vi "Measure vs B2Dv9.vi"() -> ()   [LabVIEW 2009]
doc: "This VI is an example operator panel.\n\nThe VI contains a table for the field values that may be configured manually, or loaded by checking the \"Prompt for File\" box. The data file should contain 3 columns of data, with each column delimited by a tab character.\n\nBefore the VI is executed, set the desired field units and coordinate system. Once the VI is started, follow the directions in the STATUS indicator to operate. Once a field value is achieved, it will be held indefinitely with no user intervention.\n\nThe present field is displayed in the selected units and coordinate system. The present field is queried once per second.\n\nIf a field point is specified that is outside the limits for the magnet, the VI will abort execution."
uses:
  <vilib>/Utility/file.llb/Read From Spreadsheet File (DBL).vi
panel:
  in  "go to zero at end of measurement":bool=TRUE
  in  "AH (2500)":bool=TRUE
  out "fieldvalues":string[](array[string])=["0.5", "91"]
  in  "Nr. of Accumulations":i32=3
  out "appended array":dbl[](array[numeric])=[3.9998302517106903, 162.36209894569686, 0.0, 0.0, 0.0, 0.0, 0.0, 0.0, 0.0, 0.0, 13.342744999999999, 0.0, 0.0, 3409919392.4083776]
  in  "X Axis":enum16{"B", "phi"}(ring)=enum."phi"
  in  "Y Axis":T1(ring)=enum."HP (V)"
  out "XY Graph":T2(graph)={"measured data"=[130.77697934473076, 131.17238359064999, 131.57493282279165, 131.97089096284472, 132.3709005627829, 132.7747269835502, 133.17115299337118, 133.57699453159358, 133.97291907281786, 134.37163450772164, 134.7728190578919, 135.17563033959266, 135.57333372461295, 135.97830344291987, 136.37202071047088, 136.77617688548457, 137.17728611854096, 137.57344246367185, 137.96927398938195, 138.37484712631183, 138.7678966828463, 139.1744152195974, 139.5694101008014, 139.9620548045032, 140.3756352936819, 140.76443013035026, 141.1688823561444, 141.56815184223575, 141.9675976417151, 142.3659953584458, 142.775676716873, 143.16379154430956, 143.57809589273134, 143.96940395419173, 144.37063731617485, 144.76393855420042, 145.16100725100878, 145.5613313376955, 145.9608116195239, 146.37481274459287, 146.76791709360782, 147.16896149127172, 147.5663143604346, 147.9678028289989, 148.36962760092925, 148.76598884997566, 149.16767338072717, 149.56607764958403, 149.95999407346423, 150.3722468362733, 150.76361618206533, 151.15525055318153, 151.57358356130908, 151.9672547235955, 152.360163563412, 152.76137159791082, 153.15948892689605, 153.56793804327447, 153.9626908891637, 154.35791457944399, 154.76495537165297, 155.1633906497064, 155.56156935652382, 155.96111561211768, 156.36610319740612, 156.76559958179956, 157.17093878264262, 157.56689125105595, 157.96437052200662, 158.376205209266, 158.76161261329872, 159.16724590816438, 159.55971274891448, 159.96783078495864, 160.36059978391282, 160.75915896709176, 161.17541940848784, 161.56387349300712, 161.96414973052572, 162.36209894569686], "measured data"=[47.8127675, 47.3142275, 46.9315925, 46.6304225, 46.0396825, 45.6777125, 45.4570175, 45.070972499999996, 44.789265, 44.3558025, 43.6591325, 43.409885, 43.162465, 42.71473, 42.531679999999994, 42.226214999999996, 41.899212500000004, 41.3661625, 41.03545, 40.637135, 40.367885, 40.046705, 39.865300000000005, 39.57427, 39.035422499999996, 38.758669999999995, 38.5814575, 38.362825, 37.764005, 37.63395250000001, 37.1175925, 15.572479999999999, -4.558832499999999, -4.02452, 18.98894, -4.1475925, -5.032675, 25.0248675, 27.1825925, 28.551062500000004, 27.772665, 26.5350725, 23.5985575, 27.104, 24.8567975, 23.797494999999998, 25.486569999999997, 24.9155175, 26.26794, 24.482997499999996, 25.039457499999997, 13.34384, 13.3442075, 13.3447275, 13.34462, 13.344155, 54.256817500000004, 13.3434, 13.3445175, 13.343632500000002, 13.3429575, 13.343734999999999, 13.3441525, -7.896862499999999, 13.344205, -8.8820475, 13.343815, 13.3419875, -24.604432499999998, 13.342722499999999, -6.686962499999998, 13.34337, 13.343815, 13.344335000000001, -23.786430000000003, 13.34392, 13.343657499999999, 13.3431125, 13.3426425, 13.342744999999999]}
  in  "GPIB HP 2":string="13"
  in  "Wait between \nVectors":bool=TRUE
  in  "Change\nPID\n(polar coordinates)":bool
  in  "Wait between \nVectors (ms)":u32=4000
  out "measured data":dbl[][](array[numeric])
  in  "Notes:":string="Datum: 6.04.12, Uhrzeit: 12:30,  T 4K,Winkelsweep 1° Winkelschritte, warten bei jedem Feldpunkt (measurevsB2Dv9.vi))4s, vectorsm1.txt, praktikumsprobenstab, Sweep  0.15, CrB auf CuBe Sensoren" caption="Notizen:"
  out "Messfile Refnum":refnum<file>
  in  "Measurement File":path=path "D:/UserData/Matthias/Messungen/CrB/120406/CrB_120406_anglesweep4K1.txt"
  in  "Sample name:":string="CrB"
  in  "HP 1":bool
  in  "GPIB HP":string="14"
  in  "HP 2":bool
  in  "LI 3":bool
  in  "GPIB L 3":string="8"
  in  "LI 2":bool
  in  "GPIB L 2":string="8"
  in  "LI 1":bool
  in  "GPIB L 1":string="8"
  out "Number of lines":i32=2
  in  "Operation":u16(ring)=1 items=["Stepwise", "Continous"]
  out "Ramp Rate along Vector (T/min)":dbl=0.15 format="%.3f"
  out "Current Ramp Rate Z (T/min)":dbl=0.015702717677741673 format="%.3f"
  out "Current Ramp Rate Y (T/min)":dbl=0.1491758179382072 format="%.3f"
  in  "User defined Ramp Rate (T/min)":bool=TRUE
  in  "User defined Ramp Rate (T/min)":dbl=0.15 format="%.3f"
  in  "Z-Axis Communications Config":T3={"GPIB address"=22, "GPIB bus"=1, "connection ID"=refnum, "IP"="111.111.111.1", "Active Comm Interface"=0, "Serial Port"="", "Programmer Type"=0} {"Programmer Type" items=["Model 430", "Model 420"]; "Active Comm Interface" items=["TCP/IP (Model 430 Only)", "RS232", "IEEE488"]}
  in  "Max Ramp Rate - Y Axis (A/s)":dbl=0.055 format="%.3f"
  in  "Max Ramp Rate - Z Axis (A/s)":dbl=0.19 format="%.3f"
  in  "Magnitude Limit (kG)":dbl=45.1 format="%.3f"
  in  "Y-Axis Communications Config":T3={"GPIB address"=22, "GPIB bus"=1, "connection ID"=refnum, "IP"="111.111.111.2", "Active Comm Interface"=0, "Serial Port"="", "Programmer Type"=0} {"Programmer Type" items=["Model 430", "Model 420"]; "Active Comm Interface" items=["TCP/IP (Model 430 Only)", "RS232", "IEEE488"]}
  out "Cartesian Display (T)":T4={"Y-Axis Field (T)"=0.01746, "Z-Axis Field (T)"=0.99986} {"Z-Axis Field (T)" format="%.3f"; "Y-Axis Field (T)" format="%.3f"}
  in  "Starting index":i32=1
  in  "Normal color":u32(colorbox)=11711154
  in  "Highlight color":u32(colorbox)=16711680
  in  "Prompt for File?":bool
  out "Continue Execution?":bool=TRUE
  out "error out":T5
  in  "error in":T5
  out "STATUS":string="Ramping to field vector 1..."
  in  "Ramping Control":u16(ring)=1 items=["NEXT VECTOR", "RAMPING", "HOLDING", "PAUSE", "ZERO"]
  out "Cartesian Display (kG)":T6 {"Z-Axis Field (kG)" format="%.3f"; "Y-Axis Field (kG)" format="%.3f"}
  in  "Field Values":string[][](table)=[["0.5", "90"], ["0.5", "91"]]
  out "Switch Heaters":bool=TRUE
  out "Polar Display (T)":T7={"q (degrees)"=89.97708168941708, "Field Magnitude (T)"=0.5000000399999984} {"Field Magnitude (T)" format="%.3f"; "q (degrees)" format="%.3f"}
  out "Polar Display (kG)":T8 {"Field Magnitude (kG)" format="%.3f"; "q (degrees)" format="%.3f"}
  in  "Coordinate System":u16(ring)=1 items=["Cartesian", "Polar"]
  in  "Magnetic Field Units":u16(ring)=1 items=["kG", "Tesla"]
  # "Punkt für Punkt Messung, gotozero am Ende der Messung und switch heater off"
  # "Measurement Display"
  # "Measurement Settings"
  # "Magnet Settings"
  # "Max Ramp Rate z: 1.27 T/min\nMax Ramp Rate y: 0.17 T/min"
  # "Devices"
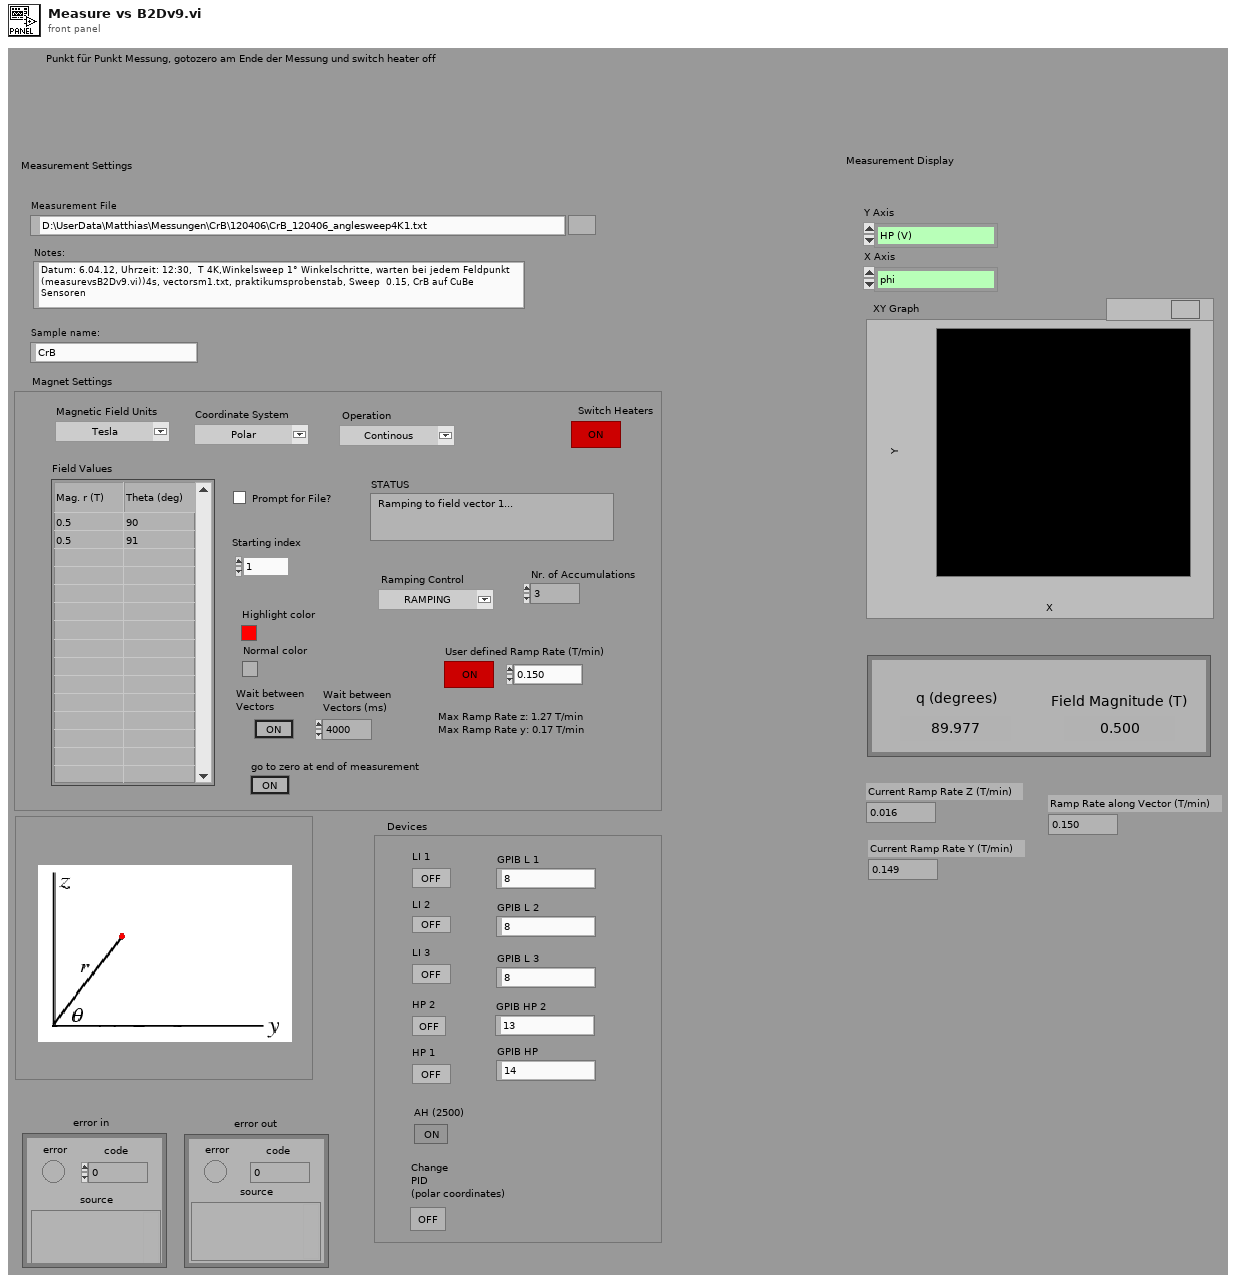
[diagram p1: front panel]
types:
  T1 = enum16{"B", "phi", "LI 1 Vx", "LI 1 phase", "LI 2 Vx", "LI 2 phase", "LI 3 Vx", "LI 3 phase", "LI 4 Vx", "LI 4 phase", "HP (V)", "AH C (pF)", "AH loss"}
  T2 = cluster{"measured data":dbl[], "measured data":dbl[]}
  T3 = cluster{"GPIB address":i16, "GPIB bus":i16, "connection ID":refnum<k5>, "IP":string, "Active Comm Interface":u16, "Serial Port":refnum<visa-resource-name>, "Programmer Type":u16}
  T4 = cluster{"Y-Axis Field (T)":dbl, "Z-Axis Field (T)":dbl}
  T5 = cluster{"error":bool, "code":i32, "source":string}
  T6 = cluster{"Y-Axis Field (kG)":dbl, "Z-Axis Field (kG)":dbl}
  T7 = cluster{"q (degrees)":dbl, "Field Magnitude (T)":dbl}
  T8 = cluster{"q (degrees)":dbl, "Field Magnitude (kG)":dbl}
  T9 = enum16{"", "RAMPING", "HOLDING", "PAUSED", "MANUAL UP", "MANUAL DOWN", "ZEROING CURRENT", "QUENCH DETECTED", "HEATING SWITCH"}
  T10 = enum16{"", "RAMPING", "HOLDING", "PAUSED", "MANUAL UP", "MANUAL DOWN", "ZEROING CURRENT", "QUENCH DETECTED", "HEATING SWITCH", "AT ZER0", "COOLING SWITCH"}
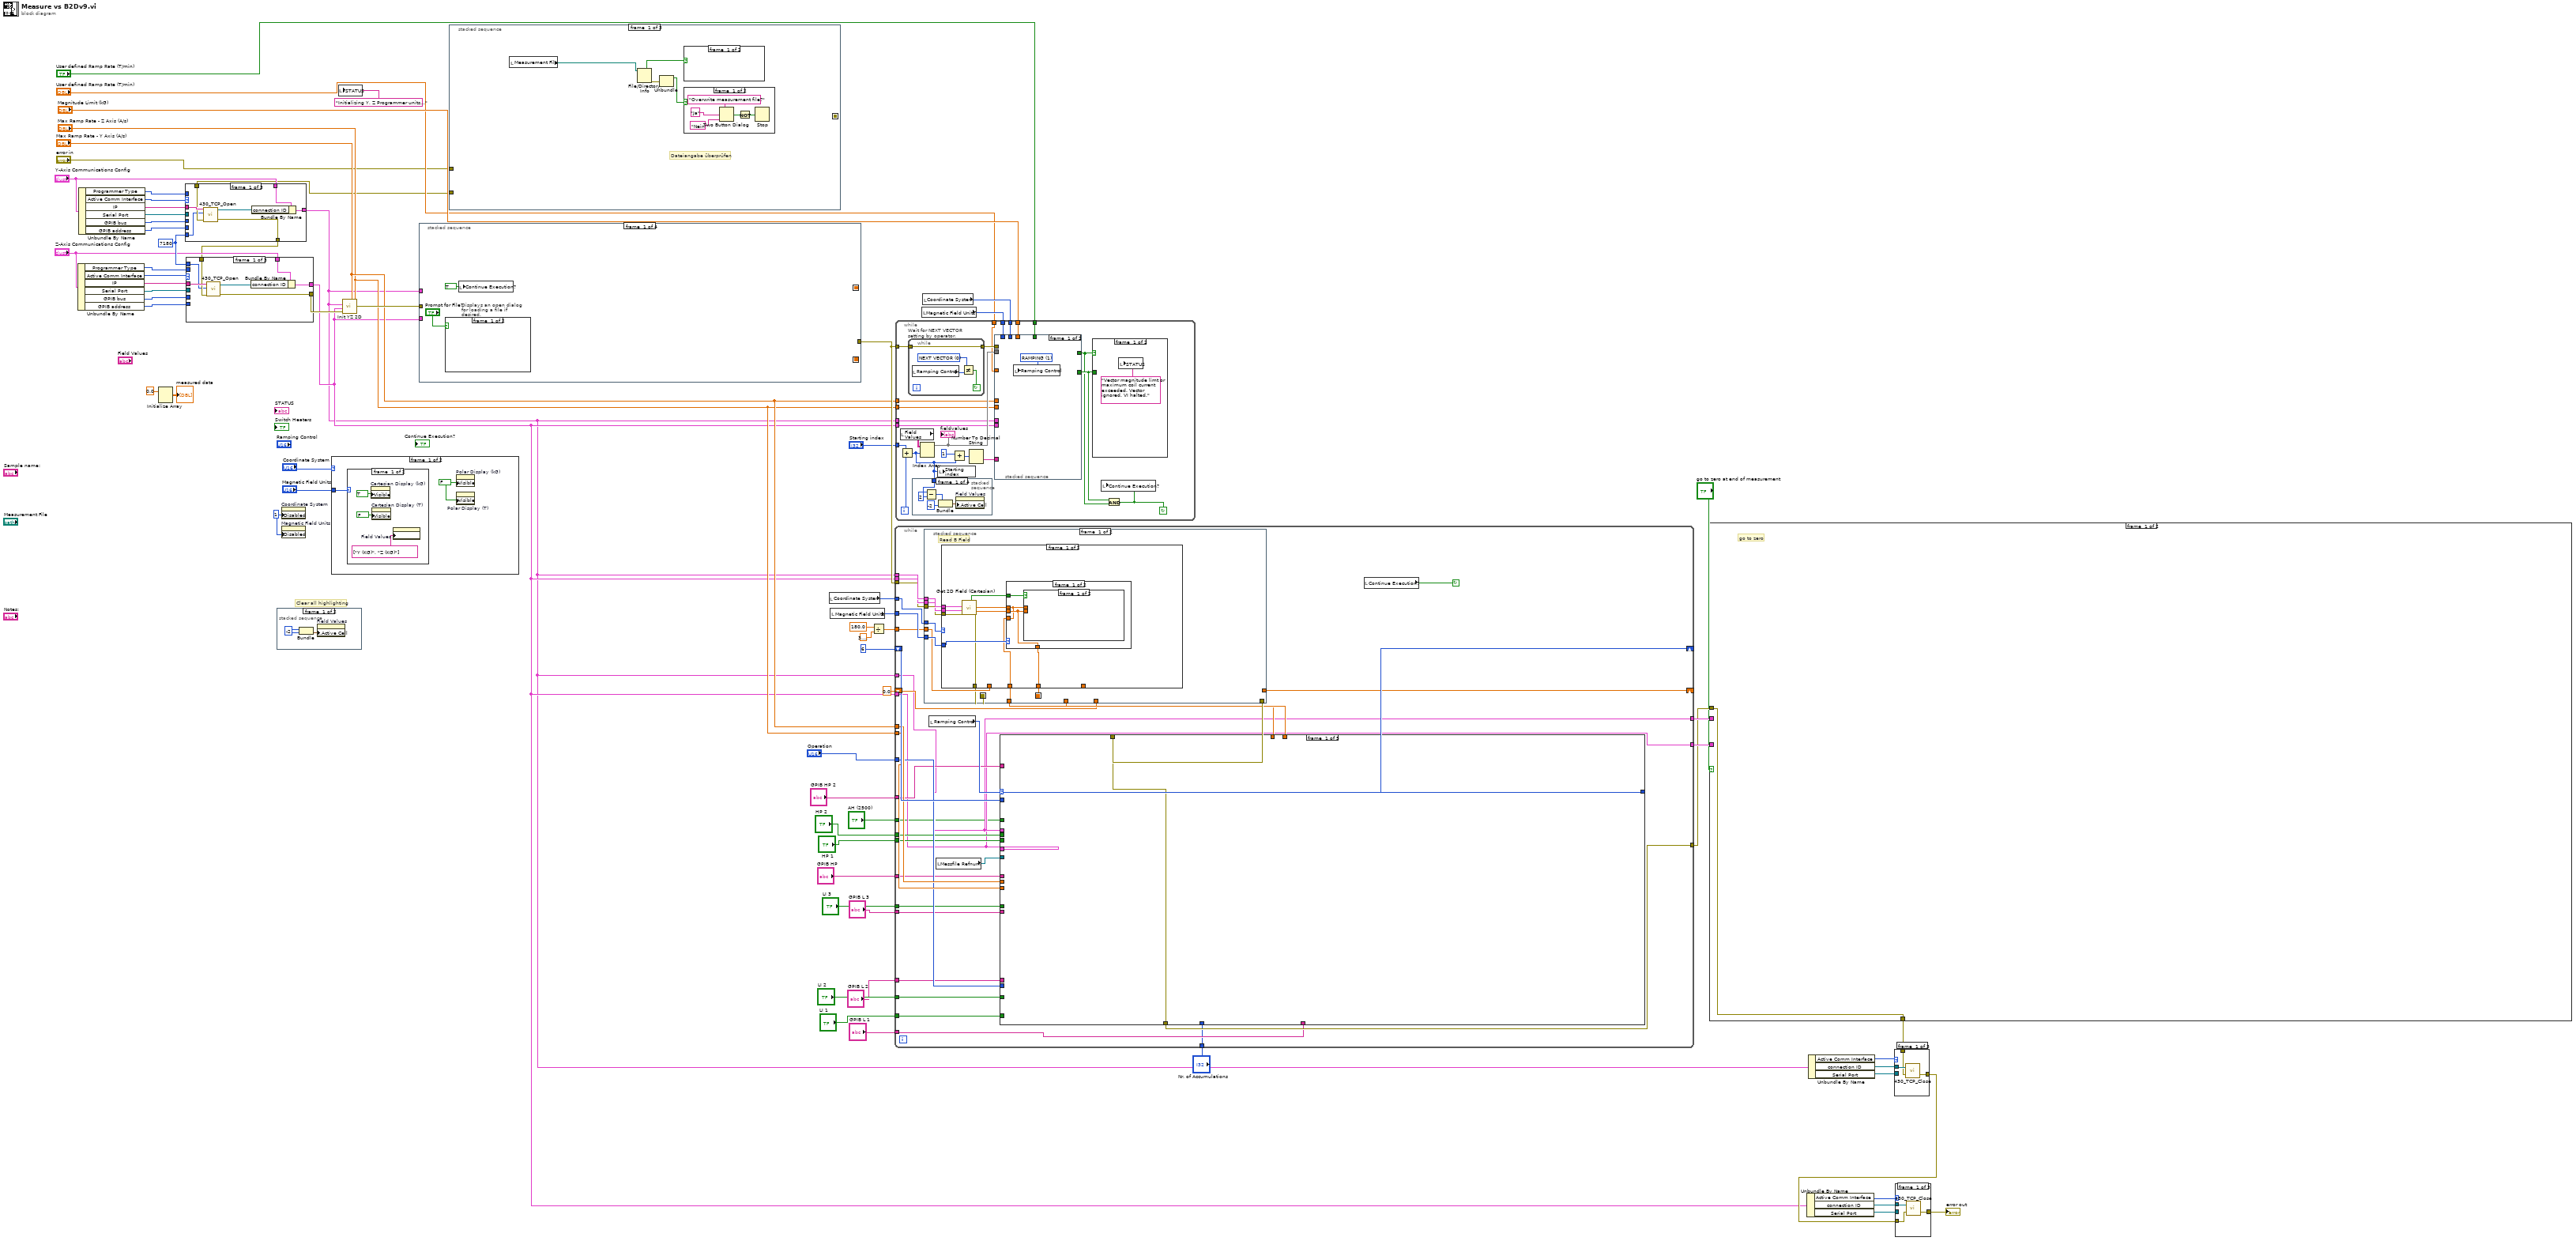
[diagram p0: block diagram]
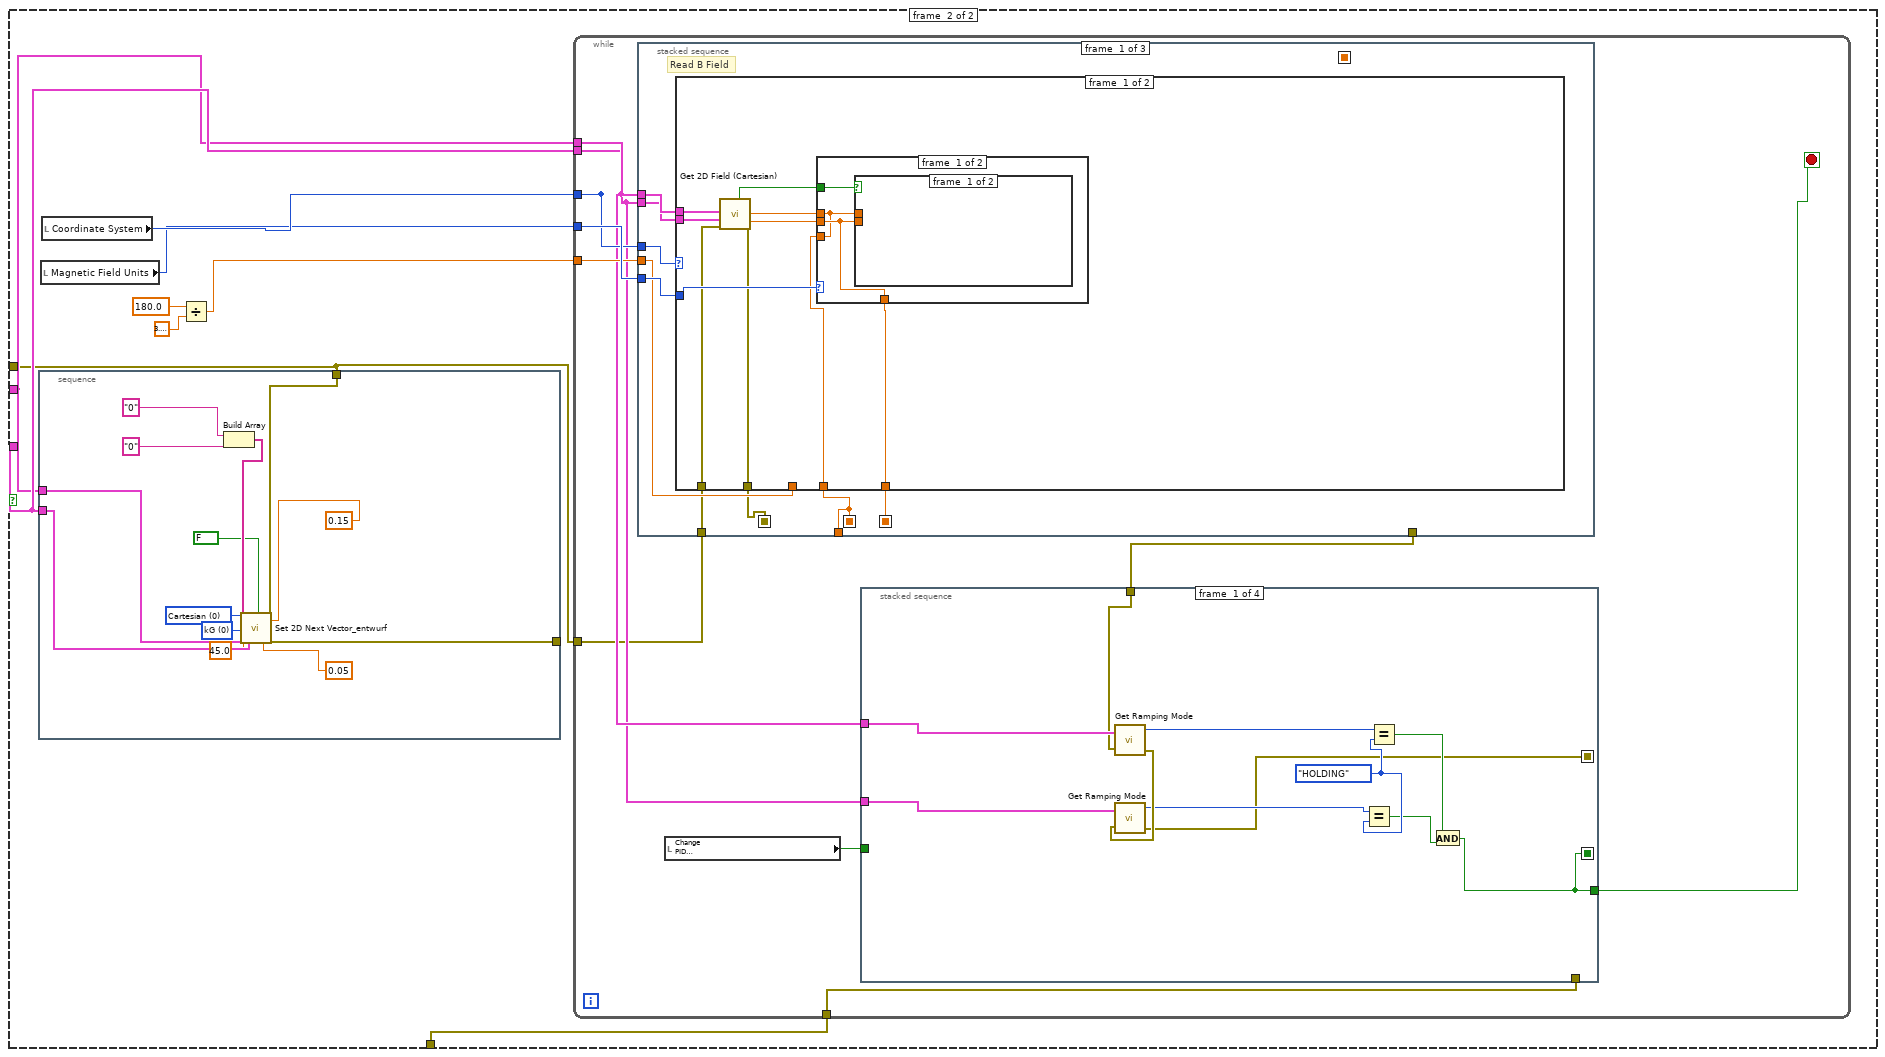
[diagram p2: hidden frame]
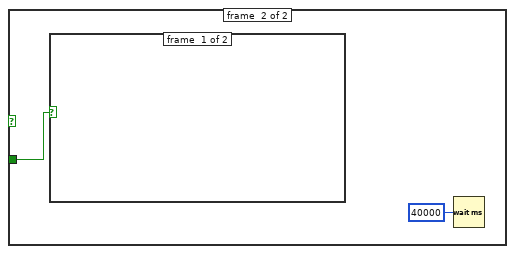
[diagram p4: hidden frame]
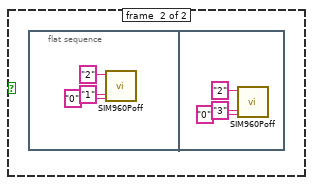
[diagram p5: hidden frame]
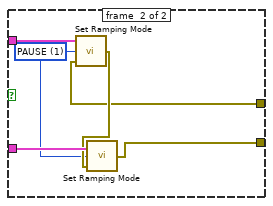
[diagram p7: hidden frame]
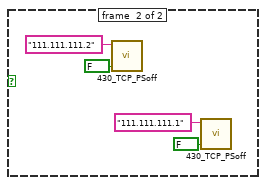
[diagram p9: hidden frame]
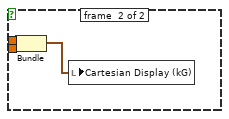
[diagram p10: hidden frame]
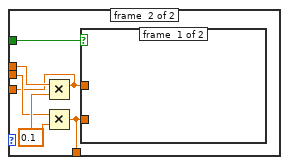
[diagram p11: hidden frame]
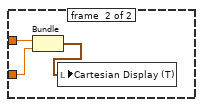
[diagram p12: hidden frame]
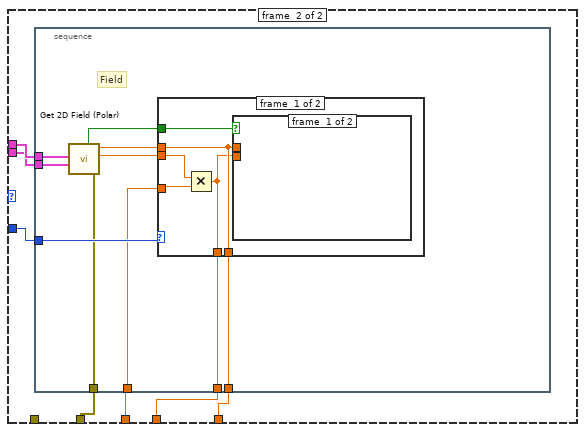
[diagram p13: hidden frame]
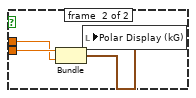
[diagram p14: hidden frame]
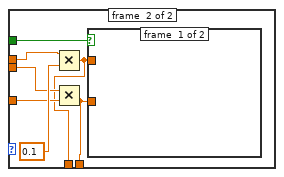
[diagram p15: hidden frame]
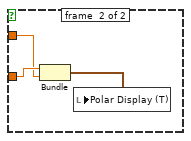
[diagram p16: hidden frame]
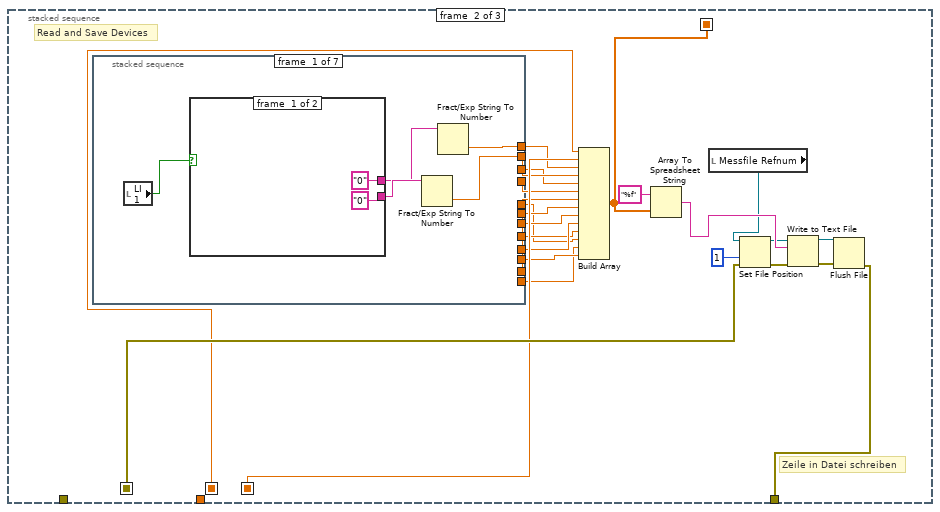
[diagram p17: hidden frame]
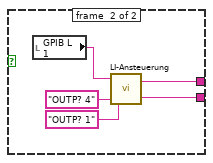
[diagram p18: hidden frame]
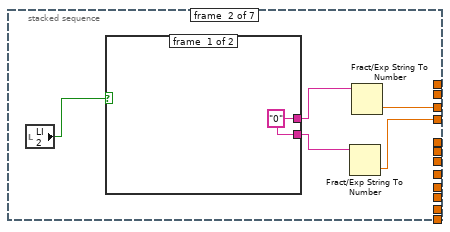
[diagram p19: hidden frame]
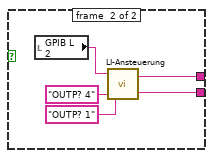
[diagram p20: hidden frame]
diagram:
  w55 = 7180 ("TCP Port")
  w68 = u8 1 ("Write Attribute")
  # "Clear all highlighting"
  n1 = Unbundle By Name("Z-Axis Communications Config") -> ("Programmer Type"=w34:u16, "Active Comm Interface"=w54:u16, "IP"=w51:string, "Serial Port"=w50:refnum<visa-resource-name>, "GPIB bus"=w33:i16, "GPIB address"=w32:i16)
  n2 = Unbundle By Name("Y-Axis Communications Config") -> ("Programmer Type"=w28:u16, "Active Comm Interface"=w53:u16, "IP"=w52:string, "Serial Port"=w49:refnum<visa-resource-name>, "GPIB bus"=w29:i16, "GPIB address"=w30:i16)
  n3 = Initialize Array(0.0 ("element")) -> (→"measured data":dbl[][])  [unwired: 2 in]
  n4 = stacked-sequence {
    frame #0 {
      w71 = -2
      n5 = Bundle(w71, w71) -> (w72:cluster{i32, i32})  [unwired: 1 in]
      n6 = property on="Field Values" class="Tbl (strict)"("Active Cell:Active Cell"=w72) -> ()  [unwired: 2 in, 2 out]
    }
    frame #1 {
      n7 = property on="Field Values" class="Tbl (strict)"("Active Cell:Cell Background Color"="Normal color") -> ()  [unwired: 2 in, 2 out]
    }
  }
  n8 = property on="Coordinate System" class="Ring (strict)"("Disabled"=w68) -> ()  [unwired: 2 in, 2 out]
  n9 = property on="Magnetic Field Units" class="Ring (strict)"("Disabled"=w68) -> ()  [unwired: 2 in, 2 out]
  n10 = case shown="0, Default" "Coordinate System" {
    tunnel: "Magnetic Field Units" -> [w75 w83]
    frame #0 {
      w74 = FALSE ("Write Attribute")
      (unwired) FALSE ("Write Attribute")
      (unwired) TRUE ("Write Attribute")
      n11 = case shown="1" w75 {
        frame #0 {
          n12 = property on="Cartesian Display (kG)" class="Cluster (strict)"("Visible"=TRUE ("Write Attribute")) -> ()  [unwired: 2 in, 2 out]
          n13 = property on="Cartesian Display (T)" class="Cluster (strict)"("Visible"=FALSE ("Write Attribute")) -> ()  [unwired: 2 in, 2 out]
          n14 = property on="Field Values" class="Tbl (strict)"("Column Header Strings[]"=string[] ["Y (KG)", "Z (KG)"] ("Write Attribute")) -> ()  [unwired: 2 in, 2 out]
        }
        frame #1 {
          n15 = property on="Cartesian Display (kG)" class="Cluster (strict)"("Visible"=FALSE ("Write Attribute")) -> ()  [unwired: 2 in, 2 out]
          n16 = property on="Cartesian Display (T)" class="Cluster (strict)"("Visible"=TRUE ("Write Attribute")) -> ()  [unwired: 2 in, 2 out]
          n17 = property on="Field Values" class="Tbl (strict)"("Column Header Strings[]"=string[] ["Y (T)", "Z (T)"] ("Write Attribute")) -> ()  [unwired: 2 in, 2 out]
        }
      }
      n18 = property on="Polar Display (kG)" class="Clust (strict)"("Visible"=w74) -> ()  [unwired: 2 in, 2 out]
      n19 = property on="Polar Display (T)" class="Clust (strict)"("Visible"=w74) -> ()  [unwired: 2 in, 2 out]
    }
    frame #1 {
      (unwired) FALSE ("Write Attribute")
      (unwired) TRUE ("Write Attribute")
      w82 = FALSE ("Write Attribute")
      n20 = case shown="1" w83 {
        frame #0 {
          n21 = property on="Polar Display (kG)" class="Clust (strict)"("Visible"=TRUE ("Write Attribute")) -> ()  [unwired: 2 in, 2 out]
          n22 = property on="Polar Display (T)" class="Clust (strict)"("Visible"=FALSE ("Write Attribute")) -> ()  [unwired: 2 in, 2 out]
          n23 = property on="Field Values" class="Tbl (strict)"("Column Header Strings[]"=string[] ["Mag. r (KG)", "Theta (deg)"] ("Write Attribute")) -> ()  [unwired: 2 in, 2 out]
        }
        frame #1 {
          n24 = property on="Polar Display (kG)" class="Clust (strict)"("Visible"=FALSE ("Write Attribute")) -> ()  [unwired: 2 in, 2 out]
          n25 = property on="Polar Display (T)" class="Clust (strict)"("Visible"=TRUE ("Write Attribute")) -> ()  [unwired: 2 in, 2 out]
          n26 = property on="Field Values" class="Tbl (strict)"("Column Header Strings[]"=string[] ["Mag. r (T)", "Theta (deg)"] ("Write Attribute")) -> ()  [unwired: 2 in, 2 out]
        }
      }
      n27 = property on="Cartesian Display (kG)" class="Cluster (strict)"("Visible"=w82) -> ()  [unwired: 2 in, 2 out]
      n28 = property on="Cartesian Display (T)" class="Cluster (strict)"("Visible"=w82) -> ()  [unwired: 2 in, 2 out]
    }
  }
  n29 = local write "STATUS"("Initializing Y, Z Programmer units..." ("STATUS")) -> ()
  n30 = stacked-sequence {
    seq-local: [_ w101 _] -> [_ _ w125]
    tunnel: "error in" -> [_ w102 _]
    tunnel: [_ _ w124] -> w23
    frame #0 {
      # "Dateiangabe überprüfen"
      n31 = local read "Measurement File"() -> (w93:path)
      n32 = File/Directory Info(path=w93) -> (directory=w91:bool, error out=w92:errorcluster)  [unwired: 1 in, 5 out]
      n33 = Unbundle(w92) -> ("status"=w90:bool)  [unwired: 2 out]
      n34 = case shown="False" w91 {
        frame #0 {
        }
        frame #1 {
          n35 = One Button Dialog(message="Invalid\nfilename!") -> (true=w99:bool)  [unwired: 1 in]
          n36 = Stop(stop? (T)=w99) -> ()
        }
      }
      n37 = case shown="False" w90 {
        frame #0 {
          n38 = Two Button Dialog(message="Overwrite measurement file?", 1:"Nein", 2:"Ja") -> (T button?=w95:bool)
          n39 = Not(x=w95) -> (.not. x?=w94:bool)
          n40 = Stop(stop? (T)=w94) -> ()
        }
        frame #1 {
        }
      }
    }
    frame #1 {
      w105 = "\r"
      # "Erstellen\ndes Headers"
      n41 = local read "User defined Ramp Rate (T/min)"() -> (w104:dbl)
      n42 = local read "Sample name:"() -> (w111:string)
      n43 = local read "Notes:"() -> (w113:string)
      n44 = Get Date/Time In Seconds() -> (seconds since 1Jan1904=w107:timestamp)
      n45 = Get Date/Time String(seconds (now)=w107) -> (date string=w109:string)  [unwired: 2 in, 1 out]
      n46 = Number To Fractional String(number=w104) -> (F-format string=w103:string)  [unwired: 3 in]
      n47 = Concatenate Strings("Date: ", w109, w105, "Sample name: ", w111, w105, "Notes: ", w113, w105, "Sweeprate: ", w103, w105) -> (w117:string)
      n48 = local read "Measurement File"() -> (w114:path)
      n49 = Open/Create/Replace File(file path (use dialog)=w114, error in=w102, operation (0:open)=4) -> (refnum out=w116:refnum<file>, error out=w118:errorcluster)  [unwired: 3 in, 1 out]
      "Messfile Refnum" <- w116
      n50 = Write to Text File(file (use dialog)=w116, text=w117, error in=w118) -> (error out=w101:errorcluster)  [unwired: 1 in, 2 out]
    }
    frame #2 {
      w121 = "\t"
      w119 = "\r"
      # "Erstellen der Spalten-\nbeschriftungen"
      n51 = local read "Messfile Refnum"() -> (w132:refnum<file>)
      n52 = Set File Position(refnum=w132, from (0:start)=1, error in=w125) -> (refnum out=w138:refnum<file>, error out=w140:errorcluster)  [unwired: 1 in]
      n53 = Concatenate Strings(w119, "B-Field Y/R", w121, "B-Field Z/phi", w121, "LI 1 Vx", w121, "LI 1 Vy", w121, "LI 2 Vx", w121, "LI 2 Vy", w121, "LI 3 Vx", w121, "LI 3 Vy", w121, "LI 4 Vx", w121, "LI 4 Vy", w121, "HP (V)", w121, w121, "AH C (pF)" ("string"), w121, "AH loss" ("string"), w121, "Timestamp", w119) -> (w139:string)
      n54 = Write to Text File(file (use dialog)=w138, text=w139, error in=w140) -> (refnum out=w142:refnum<file>, error out=w141:errorcluster)  [unwired: 1 in, 1 out]
      n55 = Flush File(refnum=w142, error in=w141) -> (error out=w124:errorcluster)  [unwired: 1 out]
    }
  }
  n56 = case shown="2" w53 {
    tunnel: w52 -> [w150 _ _]
    tunnel: w23 -> [w149 w156 w158]
    tunnel: "Y-Axis Communications Config" -> [w148 w151 w162]
    tunnel: [w146 w154 w162] -> w7
    tunnel: [w145 w155 w157] -> w31
    tunnel: w55 -> [w144 _ _]
    tunnel: w49 -> [_ w152 _]
    tunnel: w30 -> [_ _ w161]
    tunnel: w29 -> [_ _ w160]
    tunnel: w28 -> [_ _ w159]
    frame #0 {
      n57 = call <userlib>:"430_TCP_Open.vi"("IP Address"=w150, "TCP Port"=w144, "error in (no error)"=w149) -> ("connection ID"=w147:refnum<k5>, "error out"=w145:errorcluster)  [unwired: 3 in, 1 out]
      n58 = Bundle By Name(cluster=w148, "connection ID"=w147) -> (w146:T3)
    }
    frame #1 {
      n59 = call <userlib>:"430_RS232_Open.vi"("VISA resource name"=w152, "error in (no error)"=w156) -> ("VISA resource name out"=w153:refnum<visa-resource-name>, "error out"=w155:errorcluster)  [unwired: 5 in]
      n60 = Bundle By Name(cluster=w151, "Serial Port"=w153) -> (w154:T3)
    }
    frame #2 {
      n61 = case shown="0, Default" w159 {
        tunnel: w160 -> [w166 _]
        tunnel: w161 -> [w165 _]
        tunnel: w158 -> [w164 w167]
        tunnel: [w163 w167] -> w157
        frame #0 {
          n62 = DevClear(2:w164, 3:w165, 4:w166) -> (0:w163:errorcluster)  [unwired: 1 out]
        }
        frame #1 {
        }
      }
    }
  }
  n63 = case shown="2" w54 {
    tunnel: w51 -> [w174 _ _]
    tunnel: w31 -> [w173 w180 w182]
    tunnel: [w172 w179 w181] -> w48
    tunnel: "Z-Axis Communications Config" -> [w171 w177 w186]
    tunnel: [w169 w178 w186] -> w8
    tunnel: w55 -> [w168 _ _]
    tunnel: w50 -> [_ w175 _]
    tunnel: w34 -> [_ _ w185]
    tunnel: w33 -> [_ _ w184]
    tunnel: w32 -> [_ _ w183]
    frame #0 {
      n64 = call <userlib>:"430_TCP_Open.vi"("IP Address"=w174, "TCP Port"=w168, "error in (no error)"=w173) -> ("connection ID"=w170:refnum<k5>, "error out"=w172:errorcluster)  [unwired: 3 in, 1 out]
      n65 = Bundle By Name(cluster=w171, "connection ID"=w170) -> (w169:T3)
    }
    frame #1 {
      n66 = call <userlib>:"430_RS232_Open.vi"("VISA resource name"=w175, "error in (no error)"=w180) -> ("VISA resource name out"=w176:refnum<visa-resource-name>, "error out"=w179:errorcluster)  [unwired: 5 in]
      n67 = Bundle By Name(cluster=w177, "Serial Port"=w176) -> (w178:T3)
    }
    frame #2 {
      n68 = case shown="0, Default" w185 {
        tunnel: w184 -> [w190 _]
        tunnel: w183 -> [w189 _]
        tunnel: w182 -> [w188 w191]
        tunnel: [w187 w191] -> w181
        frame #0 {
          n69 = DevClear(2:w188, 3:w189, 4:w190) -> (0:w187:errorcluster)  [unwired: 1 out]
        }
        frame #1 {
        }
      }
    }
  }
  n70 = call <userlib>:"Init YZ 2D.vi"("Max Ramp Rate Z-axis"="Max Ramp Rate - Z Axis (A/s)", "Max Ramp Rate Y-axis"="Max Ramp Rate - Y Axis (A/s)", "error in"=w48, "Z-Axis Communications Config"=w8, "Y-Axis Communications Config"=w7) -> ("error out"=w66:T5)  [unwired: 5 in]
  n71 = stacked-sequence {
    seq-local: [_ w199 _ _] -> [_ _ w246 _]
    seq-local: [_ w198 _ _] -> [_ _ w245 _]
    tunnel: w8 -> [_ w201 _ _]
    tunnel: w66 -> [_ w202 _ _]
    tunnel: [_ w197 _ _] -> w62
    tunnel: w7 -> [_ w200 _ _]
    frame #0 {
      n72 = case "Displays an open dialog for loading a file if desired." shown="True" "Prompt for File?" {
        frame #0 {
        }
        frame #1 {
          n73 = call-poly <vilib>:"Read From Spreadsheet File.vi"() -> ("all rows"=w196:dbl[][])  [unwired: 7 in, 4 out]
          n74 = Number To Fractional String(number=w196, precision (6)=i16 4) -> (F-format string=w195:string[][])  [unwired: 2 in]
          n75 = local write "Field Values"(w195) -> ()
        }
      }
      n76 = local write "Continue Execution?"(TRUE ("Continue Execution?")) -> ()
    }
    frame #1 {
      w210 = u16 3 items=["NEXT VECTOR", "RAMPING", "HOLDING", "PAUSE", "ZERO"] ("Ramping Control")
      n77 = call <userlib>:"Get Switch Present.vi"("error in"=w202, "Communications Config"=w200) -> ("error out"=w206:T5, "Switch Present?"=w207:bool)
      n78 = case shown="True" w207 {
        tunnel: w206 -> [w228 w237]
        tunnel: w200 -> [_ w230]
        tunnel: [0.0 w234] -> w198
        tunnel: [w228 w236] -> w205
        frame #0 {
        }
        frame #1 {
          n79 = call <userlib>:"Get Switch Heater Time.vi"("error in"=w237, "Communications Config"=w230) -> ("error out"=w233:T5, "Switch Heating Time (secs)"=w235:dbl)
          n80 = call <userlib>:"Get Switch Heater.vi"("error in"=w233, "Communications Config"=w230) -> ("error out"=w232:T5, "Switch Heater Indicator"=w231:bool)
          n81 = case shown="False" w231 {
            tunnel: [w242 w243] -> w236
            tunnel: w235 -> [w240 _]
            tunnel: [w240 0.0] -> w234
            tunnel: w232 -> [w238 w243]
            tunnel: w230 -> [w239 _]
            frame #0 {
              n82 = call <userlib>:"Set Switch Heater.vi"("error in"=w238, "Switch Heater Control"=TRUE, "Communications Config"=w239) -> ("error out"=w242:T5)
            }
            frame #1 {
            }
          }
        }
      }
      n83 = call <userlib>:"Get Switch Present.vi"("error in"=w205, "Communications Config"=w201) -> ("error out"=w203:T5, "Switch Present?"=w204:bool)
      n84 = case shown="True" w204 {
        tunnel: w203 -> [w211 w220]
        tunnel: w201 -> [_ w213]
        tunnel: [0.0 w217] -> w199
        tunnel: [w211 w219] -> w197
        frame #0 {
        }
        frame #1 {
          n85 = call <userlib>:"Get Switch Heater Time.vi"("error in"=w220, "Communications Config"=w213) -> ("error out"=w216:T5, "Switch Heating Time (secs)"=w218:dbl)
          n86 = call <userlib>:"Get Switch Heater.vi"("error in"=w216, "Communications Config"=w213) -> ("error out"=w215:T5, "Switch Heater Indicator"=w214:bool)
          n87 = case shown="False" w214 {
            tunnel: [w221 w226] -> w219
            tunnel: w218 -> [w224 _]
            tunnel: [w224 0.0] -> w217
            tunnel: w215 -> [w222 w226]
            tunnel: w213 -> [w223 _]
            frame #0 {
              n88 = call <userlib>:"Set Switch Heater.vi"("error in"=w222, "Switch Heater Control"=TRUE, "Communications Config"=w223) -> ("error out"=w221:T5)
            }
            frame #1 {
            }
          }
        }
      }
      n89 = local write "Ramping Control"(w210) -> ()
      n90 = local write "Switch Heaters"(TRUE ("Switch Heater Control")) -> ()
      n91 = property on="Switch Heaters" class="Boolean (strict)"("Disabled"=u8 1 ("Write Attribute")) -> ()  [unwired: 2 in, 2 out]
    }
    frame #2 {
      n92 = Max & Min(x=w246, y=w245) -> (max(x,y)=w247:dbl)  [unwired: 1 out]
      n93 = local write "STATUS"("Heating switches..." ("STATUS")) -> ()
      n94 = Add(x=w247, y=2) -> (x+y=w251:dbl)
      n95 = property on="Ramping Control" class="Ring (strict)"("Disabled"=u8 1 ("Write Attribute")) -> ()  [unwired: 2 in, 2 out]
      n96 = Multiply(x=w251, y=1000) -> (x*y=w250:dbl)
      n97 = Wait (ms)(milliseconds to wait=w250) -> ()  [unwired: 1 out]
    }
    frame #3 {
      n98 = property on="Ramping Control" class="Ring (strict)"("Disabled"=u8 0 ("Write Attribute")) -> ()  [unwired: 2 in, 2 out]
      n99 = local write "STATUS"("Ready to ramp to first vector. Set Ramping Mode to NEXT VECTOR to begin." ("STATUS")) -> ()
      n100 = local read "Field Values"() -> (w256:string[][])
      n101 = Array Size(array=w256) -> (size(s)=w255:i32[])
      n102 = Index Array(array=w255, index=0) -> (element=→"Number of lines":i32)
    }
  }
  n103 = local read "Coordinate System"() -> (w63:u16)
  n104 = local read "Magnetic Field Units"() -> (w61:u16)
  n105 = Divide(x=180.0, y=3.141592653589793) -> (x/y=w58:dbl)
  n106 = while {
    shift-left: u16 6 ("Ramping Control") -> [w284]
    shift-right: [w285] -> _
    tunnel: [w287] -> w3
    tunnel: w8 -> [w261]
    tunnel: w7 -> [w262]
    tunnel: w58 -> [w289]
    tunnel: w61 -> [w290]
    tunnel: w62 -> [w291]
    tunnel: w8 -> [w292]
    tunnel: w7 -> [w293]
    tunnel: w63 -> [w279]
    tunnel: "Max Ramp Rate - Y Axis (A/s)" -> [w283]
    tunnel: "Max Ramp Rate - Z Axis (A/s)" -> [w282]
    tunnel: "Operation" -> [w281]
    tunnel: "LI 1" -> [w276]
    tunnel: "LI 2" -> [w275]
    tunnel: "LI 3" -> [w274]
    tunnel: "HP 1" -> [w273]
    tunnel: "HP 2" -> [w272]
    tunnel: "GPIB HP" -> [w271]
    tunnel: "GPIB HP 2" -> [w270]
    tunnel: "GPIB L 1" -> [w269]
    tunnel: "GPIB L 2" -> [w268]
    tunnel: "GPIB L 3" -> [w267]
    tunnel: "Nr. of Accumulations" -> [w266]
    shift-right: [w264] -> _
    shift-left: 0.0 -> [w263]
    tunnel: [w262] -> w4
    tunnel: [w261] -> w5
    tunnel: "AH (2500)" -> [w260]
    stop <- w286 continue-if-true
    n107 = stacked-sequence {
      seq-local: [w296 _] -> [_ w369]
      seq-local: [w295 _] -> [_ w366]
      tunnel: w279 -> [w302 _]
      tunnel: w293 -> [w301 _]
      tunnel: w292 -> [w300 _]
      tunnel: w291 -> [w299 _]
      tunnel: w290 -> [w298 _]
      tunnel: w289 -> [w297 _]
      tunnel: [_ w369] -> w280
      tunnel: [_ w366] -> w277
      tunnel: [w294 _] -> w278
      tunnel: [_ w367] -> w264
      tunnel: w263 -> [_ w368]
      frame #0 {
        # "Read B Field"
        n108 = case shown="1" w302 {
          tunnel: w301 -> [w312 w336]
          tunnel: w300 -> [w311 w335]
          tunnel: w299 -> [w310 w334]
          tunnel: w298 -> [w309 w333]
          tunnel: w297 -> [_ w332]
          tunnel: [w305 w331] -> w296
          tunnel: [w304 w329] -> w295
          tunnel: [w303 w330] -> w294
          tunnel: [_ w328] -> _
          frame #0 {
            n109 = call <userlib>:"Get 2D Field (Cartesian).vi"("Y-Axis Communications Config"=w312, "Z-Axis Communications Config"=w311, "error in"=w310) -> ("All Instruments Responded?"=w306:bool, "Y-Axis Field (kG)"=w308:dbl, "Z-Axis Field (kG)"=w307:dbl, "error out"=w305:T5)  [unwired: 2 in]
            n110 = case shown="1" w309 {
              tunnel: w308 -> [w313 w321]
              tunnel: w307 -> [w314 w322]
              tunnel: w306 -> [w315 w324]
              tunnel: [w314 w320] -> w304
              tunnel: [w313 w319] -> w303
              frame #0 {
                n111 = case shown="True" w315 {
                  tunnel: w313 -> [_ w317]
                  tunnel: w314 -> [_ w316]
                  frame #0 {
                  }
                  frame #1 {
                    n112 = Bundle("Y-Axis Field (kG)"=w317, "Z-Axis Field (kG)"=w316) -> (→"Cartesian Display (kG)":T6)  [unwired: 1 in]
                  }
                }
              }
              frame #1 {
                w323 = 0.1 ("y")
                n113 = Multiply(x=w321, y=w323) -> (x*y=w319:dbl)
                n114 = Multiply(x=w322, y=w323) -> (x*y=w320:dbl)
                n115 = case shown="True" w324 {
                  tunnel: w319 -> [_ w327]
                  tunnel: w320 -> [_ w326]
                  frame #0 {
                  }
                  frame #1 {
                    n116 = Bundle(w327, w326) -> (→"Cartesian Display (T)":cluster{dbl, dbl})  [unwired: 1 in]
                  }
                }
              }
            }
          }
          frame #1 {
            n117 = stacked-sequence {
              tunnel: w336 -> [w347]
              tunnel: w335 -> [w346]
              tunnel: w334 -> [w345]
              tunnel: w333 -> [w344]
              tunnel: w332 -> [w341]
              tunnel: [w339] -> w331
              tunnel: [w337] -> w329
              tunnel: [w338] -> w330
              tunnel: [w337] -> w328
              frame #0 {
                # "Field"
                n118 = call <userlib>:"Get 2D Field (Polar).vi"("Y-Axis Communications Config"=w347, "Z-Axis Communications Config"=w346, "error in"=w345) -> ("All Instruments Responded?"=w340:bool, "Radial (r) Field (kG)"=w343:dbl, "q (radians)"=w342:dbl, "error out"=w339:T5)  [unwired: 2 in]
                n119 = case shown="1" w344 {
                  tunnel: w343 -> [w349 w361]
                  tunnel: w342 -> [w351 w360]
                  tunnel: w341 -> [w350 w359]
                  tunnel: w340 -> [w352 w358]
                  tunnel: [w348 w356] -> w337
                  tunnel: [w348 w357] -> w338
                  frame #0 {
                    n120 = Multiply(x=w351, y=w350) -> (x*y=w348:dbl)
                    n121 = case shown="False" w352 {
                      tunnel: w349 -> [_ w353]
                      tunnel: w348 -> [_ w354]
                      frame #0 {
                      }
                      frame #1 {
                        n122 = Bundle(w354, "Radial (r) Field (kG)"=w353) -> (→"Polar Display (kG)":cluster{dbl, "Radial (r) Field (kG)":dbl})  [unwired: 1 in]
                      }
                    }
                  }
                  frame #1 {
                    n123 = Multiply(x=w361, y=0.1) -> (x*y=w357:dbl)
                    n124 = Multiply(x=w360, y=w359) -> (x*y=w356:dbl)
                    n125 = case shown="True" w358 {
                      tunnel: w357 -> [_ w363]
                      tunnel: w356 -> [_ w364]
                      frame #0 {
                      }
                      frame #1 {
                        n126 = Bundle(w364, w363) -> (→"Polar Display (T)":cluster{dbl, dbl})  [unwired: 1 in]
                      }
                    }
                  }
                }
              }
            }
          }
        }
      }
      frame #1 {
        # "Change PID"
        n127 = case shown="False" "Change\nPID\n(polar coordinates)" {
          tunnel: w368 -> [_ w375]
          tunnel: [_ w371] -> w367
          tunnel: w366 -> [_ w371]
          frame #0 {
          }
          frame #1 {
            n128 = local read "fieldvalues"() -> (w372:string[])
            n129 = call "SIM960Control.vi"("New Angle"=w371, "Old angle"=w375) -> ()  [unwired: 10 in]
            n130 = Index Array(array=w372, index=1 ("Index")) -> (element=w373:string)
            n131 = Fract/Exp String To Number(string=w373) -> ()  [unwired: 3 in, 2 out]
          }
        }
      }
    }
    n132 = local read "Ramping Control"() -> (w288:u16)
    n133 = local read "Messfile Refnum"() -> (w265:refnum<file>)
    n134 = case shown="1" w288 {
      selector: w288 -> [w377 w409 w563 w567 w582]
      tunnel: w262 -> [_ w411 _ w570 w587]
      tunnel: w261 -> [_ w410 _ w569 w586]
      tunnel: [w376 w381 w562 w568 w585] -> w287
      tunnel: [w377 w409 w563 w567 w582] -> w285
      tunnel: w284 -> [_ _ _ w566 w584]
      tunnel: w283 -> [_ _ _ _ w581]
      tunnel: w282 -> [_ _ _ _ w580]
      tunnel: w281 -> [_ w401 _ _ _]
      tunnel: w280 -> [w376 w397 w562 w564 w579]
      tunnel: w278 -> [_ w394 _ _ _]
      tunnel: w277 -> [_ w393 _ _ _]
      tunnel: w276 -> [_ w392 _ _ _]
      tunnel: w275 -> [_ w391 _ _ _]
      tunnel: w274 -> [_ w390 _ _ _]
      tunnel: w273 -> [_ w389 _ _ _]
      tunnel: w272 -> [_ w388 _ _ _]
      tunnel: w271 -> [_ w387 _ _ _]
      tunnel: w270 -> [_ w386 _ _ _]
      tunnel: w269 -> [_ w385 _ _ _]
      tunnel: w268 -> [_ w384 _ _ _]
      tunnel: w267 -> [_ w383 _ _ _]
      tunnel: w266 -> [_ w380 _ _ _]
      tunnel: w265 -> [_ w379 _ _ _]
      tunnel: w260 -> [_ w378 _ _ _]
      frame #0 {
      }
      frame #1 {
        w404 = T9."HOLDING" ("y")
        n135 = local read "Number of lines"() -> (w398:i32)
        n136 = local read "Starting index"() -> (w400:i32)
        n137 = call <userlib>:"Get Ramping Mode.vi"("Communications Config"=w411, "error in"=w397) -> ("Ramping Mode"=w407:T10, "error out"=w408:T5)  [unwired: 1 out]
        n138 = call <userlib>:"Get Ramping Mode.vi"("Communications Config"=w410, "error in"=w408) -> ("Ramping Mode"=w406:T10, "error out"=w382:T5)  [unwired: 1 out]
        n139 = Less?(x=w400, y=w398) -> (x < y?=w399:bool)
        n140 = Equal?(x=w407, y=w404) -> (x = y?=w403:bool)
        n141 = Equal?(x=w406, y=w404) -> (x = y?=w402:bool)
        n142 = Compound Arithmetic op=AND(w403, w402) -> (w405:bool)
        n143 = case shown="True" w405 {
          tunnel: w401 -> [_ w433]
          tunnel: w399 -> [_ w432]
          tunnel: "Wait between \nVectors (ms)" -> [_ w431]
          tunnel: "Wait between \nVectors" -> [_ w430]
          tunnel: w394 -> [_ w429]
          tunnel: w393 -> [_ w428]
          tunnel: w392 -> [_ w427]
          tunnel: w391 -> [_ w426]
          tunnel: w390 -> [_ w425]
          tunnel: w389 -> [_ w424]
          tunnel: w388 -> [_ w423]
          tunnel: w387 -> [_ w422]
          tunnel: w386 -> [_ w421]
          tunnel: w385 -> [_ w420]
          tunnel: w384 -> [_ w419]
          tunnel: w383 -> [_ w418]
          tunnel: w382 -> [w412 w417]
          tunnel: [w412 w416] -> w381
          tunnel: w380 -> [_ w415]
          tunnel: w379 -> [_ w414]
          tunnel: w378 -> [_ w413]
          frame #0 {
          }
          frame #1 {
            n144 = case shown="1" w433 {
              tunnel: w432 -> [_ w456]
              tunnel: w431 -> [_ w455]
              tunnel: w430 -> [_ w454]
              tunnel: w429 -> [_ w453]
              tunnel: w428 -> [_ w452]
              tunnel: w427 -> [_ w451]
              tunnel: w426 -> [_ w450]
              tunnel: w425 -> [_ w449]
              tunnel: w424 -> [_ w448]
              tunnel: w423 -> [_ w447]
              tunnel: w422 -> [_ w446]
              tunnel: w421 -> [_ w445]
              tunnel: w420 -> [_ w444]
              tunnel: w419 -> [_ w443]
              tunnel: w418 -> [_ w442]
              tunnel: w417 -> [w434 w441]
              tunnel: [w434 w440] -> w416
              tunnel: w415 -> [_ w439]
              tunnel: w414 -> [_ w438]
              tunnel: w413 -> [_ w437]
              frame #0 {
                w436 = u16 2 items=["NEXT VECTOR", "RAMPING", "HOLDING", "PAUSE", "ZERO"] ("Ramping Control")
                n145 = local write "STATUS"("Holding at current vector. Set Ramping Mode to NEXT VECTOR to continue." ("STATUS")) -> ()
                n146 = local write "Ramping Control"(w436) -> ()
              }
              frame #1 {
                # "Go to NEXT VECTOR automatically"
                n147 = case shown="True" w456 {
                  tunnel: w455 -> [_ w479]
                  tunnel: w454 -> [_ w478]
                  tunnel: w453 -> [_ w477]
                  tunnel: w452 -> [_ w476]
                  tunnel: w451 -> [_ w475]
                  tunnel: w450 -> [_ w474]
                  tunnel: w449 -> [_ w473]
                  tunnel: w448 -> [_ w472]
                  tunnel: w447 -> [_ w471]
                  tunnel: w446 -> [_ w470]
                  tunnel: w445 -> [_ w469]
                  tunnel: w444 -> [_ w468]
                  tunnel: w443 -> [_ w467]
                  tunnel: w442 -> [_ w466]
                  tunnel: w441 -> [w458 w465]
                  tunnel: [w458 w464] -> w440
                  tunnel: w439 -> [_ w463]
                  tunnel: w438 -> [_ w462]
                  tunnel: w437 -> [_ w461]
                  frame #0 {
                    w460 = u16 2 items=["NEXT VECTOR", "RAMPING", "HOLDING", "PAUSE", "ZERO"] ("Ramping Control")
                    n148 = local write "STATUS"("Holding at current vector. Set Ramping Mode to NEXT VECTOR to continue." ("STATUS")) -> ()
                    n149 = local write "Ramping Control"(w460) -> ()
                    n150 = local write "Continue Execution?"(FALSE) -> ()
                  }
                  frame #1 {
                    n151 = stacked-sequence {
                      tunnel: w479 -> [w498 _]
                      tunnel: w478 -> [w497 _]
                      tunnel: w477 -> [w496 _]
                      tunnel: w476 -> [w495 _]
                      tunnel: w475 -> [w494 _]
                      tunnel: w474 -> [w493 _]
                      tunnel: w473 -> [w492 _]
                      tunnel: w472 -> [w491 _]
                      tunnel: w471 -> [w490 _]
                      tunnel: w470 -> [w489 _]
                      tunnel: w469 -> [w488 _]
                      tunnel: w468 -> [w487 _]
                      tunnel: w467 -> [w486 _]
                      tunnel: w466 -> [w485 _]
                      tunnel: w465 -> [w484 _]
                      tunnel: [w483 _] -> w464
                      tunnel: w463 -> [w482 _]
                      tunnel: w462 -> [w481 _]
                      tunnel: w461 -> [w480 _]
                      frame #0 {
                        n152 = case shown="True" w497 {
                          tunnel: w498 -> [_ w517]
                          tunnel: w496 -> [_ w516]
                          tunnel: w495 -> [_ w515]
                          tunnel: w494 -> [_ w514]
                          tunnel: w493 -> [_ w513]
                          tunnel: w492 -> [_ w512]
                          tunnel: w491 -> [_ w511]
                          tunnel: w490 -> [_ w510]
                          tunnel: w489 -> [_ w509]
                          tunnel: w488 -> [_ w508]
                          tunnel: w487 -> [_ w507]
                          tunnel: w486 -> [_ w506]
                          tunnel: w485 -> [_ w505]
                          tunnel: w484 -> [w499 w504]
                          tunnel: [w499 w503] -> w483
                          tunnel: w482 -> [_ w502]
                          tunnel: w481 -> [_ w501]
                          tunnel: w480 -> [_ w500]
                          frame #0 {
                          }
                          frame #1 {
                            n153 = stacked-sequence {
                              tunnel: w517 -> [w518 _ _]
                              tunnel: w516 -> [_ w551 _]
                              tunnel: w515 -> [_ w550 _]
                              tunnel: [_ w520 _] -> _
                              tunnel: w514 -> [_ w549 _]
                              tunnel: w513 -> [_ w548 _]
                              tunnel: w512 -> [_ w547 _]
                              tunnel: w511 -> [_ w546 _]
                              tunnel: w510 -> [_ w545 _]
                              tunnel: w509 -> [_ w544 _]
                              tunnel: w508 -> [_ w543 _]
                              tunnel: w507 -> [_ w542 _]
                              tunnel: w506 -> [_ w541 _]
                              tunnel: w505 -> [_ w540 _]
                              tunnel: w504 -> [_ w539 _]
                              tunnel: [_ w524 _] -> w503
                              tunnel: w502 -> [_ w523 _]
                              tunnel: w501 -> [_ w520 _]
                              tunnel: w500 -> [_ w519 _]
                              frame #0 {
                                n154 = Wait (ms)(milliseconds to wait=w518) -> ()  [unwired: 1 out]
                              }
                              frame #1 {
                                n155 = call "ReadallDevicesv2.vi"("GPIB HP 2"=w543, "HP 2"=w545, "AH"=w519, "GPIB HP"=w544, "HP 1"=w546, "error in"=w539, "LI 3"=w547, "GPIB L 3"=w540, "LI 2"=w548, "GPIB L 2"=w541, "LI 1"=w549, "GPIB L 1"=w542, "Nr. of Accumulations"=w523, "Y-Axis Field (kG)"=w551, "Radial (r) Field (kG) 2"=w550) -> ("appended array"=w521:dbl[], "error out"=w525:errorcluster)  [unwired: 3 in]
                                "appended array" <- w521
                                n156 = Array To Spreadsheet String(array=w521, 3:"%.9f" ("format string")) -> (spreadsheet string=w526:string)  [unwired: 1 in]
                                n157 = local read "measured data"() -> (w538:dbl[][])
                                n158 = Insert Into Array(array=w538, new element=w521) -> (w522:dbl[][])  [unwired: 2 in]
                                n159 = Index Array(array=w522, index (col)="X Axis") -> (element=w537:dbl[])  [unwired: 1 in]
                                n160 = Index Array(array=w522, index (col)="Y Axis") -> (element=w536:dbl[])  [unwired: 1 in]
                                n161 = Set File Position(refnum=w520, from (0:start)=1, error in=w525) -> (refnum out=w531:refnum<file>, error out=w530:errorcluster)  [unwired: 1 in]
                                n162 = Bundle("measured data"=w537, "measured data"=w536) -> (w535:T2)  [unwired: 1 in]
                                n163 = local write "measured data"(w522) -> ()
                                n164 = Write to Text File(file (use dialog)=w531, text=w526, error in=w530) -> (refnum out=w528:refnum<file>, error out=w529:errorcluster)  [unwired: 1 in, 1 out]
                                n165 = local write "XY Graph"(w535) -> ()
                                n166 = Flush File(refnum=w528, error in=w529) -> (error out=w524:errorcluster)  [unwired: 1 out]
                              }
                              frame #2 {
                                # "Restart PID after PID logout"
                                n167 = local read "appended array"() -> (w557:dbl[])
                                n168 = Index Array(array=w557, index=10) -> (element=w555:dbl)
                                n169 = Absolute Value(x=w555) -> (abs(x)=w554:dbl)
                                n170 = Greater Or Equal?(x=w554, y=260.0) -> (x >= y?=w552:bool)
                                n171 = case shown="True" w552 {
                                frame #0 {
                                }
                                frame #1 {
                                n172 = call "SIM960restartPID.vi"("Restart Damping"=FALSE, "GPIB-Adress"="2") -> ()  [unwired: 10 in]
                                }
                                }
                              }
                            }
                          }
                        }
                      }
                      frame #1 {
                        w561 = u16 0 items=["NEXT VECTOR", "RAMPING", "HOLDING", "PAUSE", "ZERO"] ("Ramping Control")
                        n173 = local write "Ramping Control"(w561) -> ()
                        n174 = local write "STATUS"("Go to NEXT VECTOR" ("STATUS")) -> ()
                      }
                    }
                  }
                }
              }
            }
          }
        }
      }
      frame #2 {
      }
      frame #3 {
        n175 = Not Equal?(x=w567, y=w566) -> (x != y?=w565:bool)
        n176 = case shown="True" w565 {
          tunnel: w570 -> [_ w578]
          tunnel: w569 -> [_ w577]
          tunnel: [w571 w575] -> w568
          tunnel: w564 -> [w571 w572]
          frame #0 {
          }
          frame #1 {
            w573 = u16 1 items=["RAMP", "PAUSE", "MANUAL UP", "MANUAL DOWN", "ZERO"] ("Ramping Mode")
            n177 = call <userlib>:"Set Ramping Mode.vi"("error in"=w572, "Ramping Mode"=w573, "Communications Config"=w578) -> ("error out"=w576:T5)
            n178 = call <userlib>:"Set Ramping Mode.vi"("error in"=w576, "Ramping Mode"=w573, "Communications Config"=w577) -> ("error out"=w575:T5)
            n179 = local write "STATUS"("All Programmers are PAUSED. Set Ramping Mode to NEXT VECTOR to continue." ("STATUS")) -> ()
          }
        }
      }
      frame #4 {
        n180 = Not Equal?(x=w582, y=w584) -> (x != y?=w583:bool)
        n181 = case shown="True" w583 {
          tunnel: w587 -> [_ w596]
          tunnel: w586 -> [_ w595]
          tunnel: [w588 w591] -> w585
          tunnel: w581 -> [_ w594]
          tunnel: w580 -> [_ w593]
          tunnel: w579 -> [w588 w589]
          frame #0 {
          }
          frame #1 {
            w590 = u16 4 items=["RAMP", "PAUSE", "MANUAL UP", "MANUAL DOWN", "ZERO"] ("Ramping Mode")
            n182 = local write "STATUS"("Zeroing vector." ("STATUS")) -> ()
            n183 = call <userlib>:"Set Ramping Mode.vi"("error in"=w589, "Ramping Mode"=w590, "Communications Config"=w596) -> ("error out"=w599:T5)
            n184 = call <userlib>:"Set Ramping Mode.vi"("error in"=w599, "Ramping Mode"=w590, "Communications Config"=w595) -> ("error out"=w592:T5)
            n185 = call <userlib>:"Set Current Ramp Rate.vi"("Communications Config"=w596, "Ramp Rate (A/sec)"=w594, "error in"=w592) -> ("error out"=w597:T5)  [unwired: 2 in]
            n186 = call <userlib>:"Set Current Ramp Rate.vi"("Communications Config"=w595, "Ramp Rate (A/sec)"=w593, "error in"=w597) -> ("error out"=w591:T5)  [unwired: 2 in]
          }
        }
      }
    }
    n187 = local read "Continue Execution?"() -> (w286:bool)
  }
  n188 = local read "Magnetic Field Units"() -> (w64:u16)
  n189 = local read "Coordinate System"() -> (w65:u16)
  n190 = while {
    tunnel: "Starting index" -> [w607]
    tunnel: w8 -> [w613]
    tunnel: w7 -> [w614]
    tunnel: w64 -> [w615]
    tunnel: w65 -> [w616]
    tunnel: w62 -> [w619]
    tunnel: "Max Ramp Rate - Y Axis (A/s)" -> [w603]
    tunnel: "Max Ramp Rate - Z Axis (A/s)" -> [w602]
    tunnel: "Magnitude Limit (kG)" -> [w604]
    tunnel: "User defined Ramp Rate (T/min)" -> [w601]
    tunnel: "User defined Ramp Rate (T/min)" -> [w600]
    i -> [w606]
    stop <- w608 continue-if-true
    n191 = local read "Field Values"() -> (w610:string[][])
    n192 = Add(x=w607, y=w606) -> (x+y=w605:i32)
    n193 = while "Wait for NEXT VECTOR setting by operator." {
      tunnel: [w623] -> w618
      tunnel: w619 -> [w623]
      stop <- w624 continue-if-true
      w622 = u16 0 items=["NEXT VECTOR", "RAMPING", "HOLDING", "PAUSE", "ZERO"] ("Ramping Control")
      n194 = local read "Ramping Control"() -> (w625:u16)
      n195 = Not Equal?(x=w622, y=w625) -> (x != y?=w624:bool)
    }
    n196 = stacked-sequence {
      tunnel: w605 -> [w627 _ w633 _]
      frame #0 {
        (unwired) -2
        n197 = Subtract(x=w627, y=2) -> (x-y=w630:i32)
        n198 = Bundle(w630, -2) -> (w628:cluster{i32, i32})  [unwired: 1 in]
        n199 = property on="Field Values" class="Tbl (strict)"("Active Cell:Active Cell"=w628) -> ()  [unwired: 2 in, 2 out]
      }
      frame #1 {
        n200 = local read "Normal color"() -> (w631:u32)
        n201 = property on="Field Values" class="Tbl (strict)"("Active Cell:Cell Background Color"=w631) -> ()  [unwired: 2 in, 2 out]
      }
      frame #2 {
        n202 = Decrement(x=w633) -> (x-1=w632:i32)
        n203 = Bundle(w632, -2) -> (w635:cluster{i32, i32})  [unwired: 1 in]
        n204 = property on="Field Values" class="Tbl (strict)"("Active Cell:Active Cell"=w635) -> ()  [unwired: 2 in, 2 out]
      }
      frame #3 {
        n205 = property on="Field Values" class="Tbl (strict)"("Active Cell:Cell Background Color"="Highlight color") -> ()  [unwired: 2 in, 2 out]
      }
    }
    n206 = Index Array(array=w610, index (row)=w605) -> (element=w617:string[])  [unwired: 1 in]
    "fieldvalues" <- w617
    n207 = local write "Starting index"(w605) -> ()
    n208 = Add(x=1, y=w605) -> (x+y=w620:i32)
    n209 = Number To Decimal String(number=w620) -> (decimal integer string=w609:string)  [unwired: 1 in]
    n210 = stacked-sequence {
      tunnel: [_ w661] -> w611
      tunnel: [_ w660] -> w612
      tunnel: w618 -> [_ w656]
      tunnel: w617 -> [_ w655]
      tunnel: w616 -> [_ w654]
      tunnel: w615 -> [_ w653]
      tunnel: w614 -> [_ w652]
      tunnel: w613 -> [_ w651]
      tunnel: w609 -> [_ w650]
      tunnel: w604 -> [_ w648]
      tunnel: w603 -> [_ w647]
      tunnel: w602 -> [_ w642]
      tunnel: w601 -> [_ w646]
      tunnel: w600 -> [_ w645]
      frame #0 {
        w640 = u16 1 items=["NEXT VECTOR", "RAMPING", "HOLDING", "PAUSE", "ZERO"] ("Ramping Control")
        n211 = local write "Ramping Control"(w640) -> ()
      }
      frame #1 {
        n212 = call <userlib>:"Set 2D Next Vector_entwurf.vi"("Coordinate System"=w654, "Magnetic Field Units"=w653, 3:"User defined Ramp Rate (T/min)"=w645, "Magnitude Limit (kG)"=w648, "Y-Axis Communications Config"=w652, "Input Vector"=w655, "Z-Axis Communications Config"=w651, 10:"User defined Ramp Rate (T/min)"=w646, "Max Ramp Rate - Y Axis (A/s)"=w647, "error in"=w656, "Max Ramp Rate - Z Axis (A/s)"=w642) -> ("Y-Axis Ramp Rate (T/min)"=→"Current Ramp Rate Y (T/min)":dbl, "Within Limits?"=w661:bool, "Ramp Rate along Vector (T/min)"=→"Ramp Rate along Vector (T/min)":dbl, "Z-Axis Ramp Rate (T/min)"=→"Current Ramp Rate Z (T/min)":dbl, "All Instruments Responded?"=w660:bool, "error out"=w649:T5)  [unwired: 3 in]
        n213 = Concatenate Strings("Ramping to field vector " ("STATUS"), w650, "..." ("STATUS")) -> (w657:string)
        n214 = local write "error in"(w649) -> ()
        n215 = local write "STATUS"(w657) -> ()
      }
    }
    n216 = case shown="True" w611 {
      tunnel: w612 -> [_ w638]
      frame #0 {
        n217 = local write "STATUS"("Vector magnitude limt or maximum coil current exceeded. Vector ignored. VI halted." ("STATUS")) -> ()
      }
      frame #1 {
        n218 = case shown="True" w638 {
          frame #0 {
            n219 = local write "STATUS"("Not all programmers responded. VI halted." ("STATUS")) -> ()
          }
          frame #1 {
          }
        }
      }
    }
    n220 = Compound Arithmetic op=AND(w612, w611) -> (w608:bool)
    n221 = local write "Continue Execution?"(w608) -> ()
  }
  n222 = case shown="True" "go to zero at end of measurement" {
    tunnel: [w662 w666] -> w6
    tunnel: w5 -> [_ w665]
    tunnel: w4 -> [_ w664]
    tunnel: w3 -> [w662 w663]
    frame #0 {
      # "go to zero"
    }
    frame #1 {
      n223 = stacked-sequence {
        tunnel: w664 -> [w683]
        tunnel: w665 -> [w684]
        tunnel: w663 -> [w674]
        tunnel: [w673] -> _
        frame #0 {
          w678 = u16 0 items=["kG", "Tesla"] ("Magnetic Field Units")
          w679 = u16 0 items=["Cartesian", "Polar"] ("Coordinate System")
          n224 = Build Array("0", "0") -> (w680:string[])
          n225 = call <userlib>:"Set 2D Next Vector_entwurf.vi"("Coordinate System"=w679, "Magnetic Field Units"=w678, "Magnitude Limit (kG)"=45.0, "Y-Axis Communications Config"=w683, "Input Vector"=w680, "Z-Axis Communications Config"=w684, "User defined Ramp Rate (T/min)"=FALSE, "Max Ramp Rate - Y Axis (A/s)"=0.05, "error in"=w674, "Max Ramp Rate - Z Axis (A/s)"=0.15) -> ("error out"=w673:T5)  [unwired: 4 in, 5 out]
        }
      }
      n226 = local read "Magnetic Field Units"() -> (w668:u16)
      n227 = local read "Coordinate System"() -> (w669:u16)
      n228 = Divide(x=180.0, y=3.141592653589793) -> (x/y=w667:dbl)
      n229 = while {
        tunnel: w667 -> [w693]
        tunnel: w668 -> [w694]
        tunnel: w665 -> [w690]
        tunnel: w664 -> [w691]
        tunnel: [w692] -> _
        tunnel: w669 -> [w692]
        tunnel: [w687] -> w666
        tunnel: w663 -> [w686]
        stop <- w688 stop-if-true
        n230 = stacked-sequence {
          seq-local: [w736 _ _] -> [_ w826 _]
          seq-local: [w735 _ _] -> [_ w823 _]
          seq-local: [w733 _ _] -> [_ w824 _]
          seq-local: [_ w811 _] -> [_ _ w886]
          tunnel: w692 -> [w741 _ w884]
          tunnel: w691 -> [w740 _ _]
          tunnel: w690 -> [w739 _ _]
          tunnel: w694 -> [w738 _ _]
          tunnel: w693 -> [w737 _ _]
          tunnel: [_ w825 _] -> w689
          tunnel: w686 -> [w734 _ _]
          tunnel: [w733 _ _] -> _
          frame #0 {
            # "Read B Field"
            n231 = case shown="0, Default" w741 {
              tunnel: w740 -> [w751 w773]
              tunnel: w739 -> [w750 w772]
              tunnel: w738 -> [w749 w771]
              tunnel: w737 -> [_ w770]
              tunnel: [w745 w769] -> w736
              tunnel: [w744 w767] -> w735
              tunnel: [w743 w768] -> w733
              tunnel: w734 -> [w742 _]
              frame #0 {
                n232 = call <userlib>:"Get 2D Field (Cartesian).vi"("Y-Axis Communications Config"=w751, "Z-Axis Communications Config"=w750, "error in"=w742) -> ("All Instruments Responded?"=w746:bool, "Y-Axis Field (kG)"=w748:dbl, "Z-Axis Field (kG)"=w747:dbl, "error out"=w745:T5)  [unwired: 2 in]
                n233 = case shown="1" w749 {
                  tunnel: w748 -> [w752 w760]
                  tunnel: w747 -> [w753 w761]
                  tunnel: w746 -> [w754 w763]
                  tunnel: [w753 w759] -> w744
                  tunnel: [w752 w758] -> w743
                  frame #0 {
                    n234 = case shown="False" w754 {
                      tunnel: w752 -> [_ w757]
                      tunnel: w753 -> [_ w756]
                      frame #0 {
                      }
                      frame #1 {
                        n235 = Bundle("Y-Axis Field (kG)"=w757, "Z-Axis Field (kG)"=w756) -> (w755:T6)  [unwired: 1 in]
                        n236 = local write "Cartesian Display (kG)"(w755) -> ()
                      }
                    }
                  }
                  frame #1 {
                    w762 = 0.1 ("y")
                    n237 = Multiply(x=w760, y=w762) -> (x*y=w758:dbl)
                    n238 = Multiply(x=w761, y=w762) -> (x*y=w759:dbl)
                    n239 = case shown="True" w763 {
                      tunnel: w758 -> [_ w766]
                      tunnel: w759 -> [_ w765]
                      frame #0 {
                      }
                      frame #1 {
                        n240 = Bundle(w766, w765) -> (w764:cluster{dbl, dbl})  [unwired: 1 in]
                        n241 = local write "Cartesian Display (T)"(w764) -> ()
                      }
                    }
                  }
                }
              }
              frame #1 {
                n242 = stacked-sequence {
                  tunnel: w773 -> [w783]
                  tunnel: w772 -> [w782]
                  tunnel: w771 -> [w781]
                  tunnel: w770 -> [w778]
                  tunnel: [w776] -> w769
                  tunnel: [w775] -> w767
                  tunnel: [w774] -> w768
                  frame #0 {
                    # "Field"
                    n243 = call <userlib>:"Get 2D Field (Polar).vi"("Y-Axis Communications Config"=w783, "Z-Axis Communications Config"=w782) -> ("All Instruments Responded?"=w777:bool, "Radial (r) Field (kG)"=w780:dbl, "q (radians)"=w779:dbl, "error out"=w776:T5)  [unwired: 3 in]
                    n244 = case shown="1" w781 {
                      tunnel: w780 -> [w785 w797]
                      tunnel: w779 -> [w787 w796]
                      tunnel: w778 -> [w786 w795]
                      tunnel: w777 -> [w788 w794]
                      tunnel: [w785 w792] -> w775
                      tunnel: [w784 w793] -> w774
                      frame #0 {
                        n245 = Multiply(x=w787, y=w786) -> (x*y=w784:dbl)
                        n246 = case shown="True" w788 {
                          tunnel: w785 -> [_ w790]
                          tunnel: w784 -> [_ w791]
                          frame #0 {
                          }
                          frame #1 {
                            n247 = Bundle(w791, "Radial (r) Field (kG)"=w790) -> (w789:cluster{dbl, "Radial (r) Field (kG)":dbl})  [unwired: 1 in]
                            n248 = local write "Polar Display (kG)"(w789) -> ()
                          }
                        }
                      }
                      frame #1 {
                        n249 = Multiply(x=w797, y=0.1) -> (x*y=w793:dbl)
                        n250 = Multiply(x=w796, y=w795) -> (x*y=w792:dbl)
                        n251 = case shown="True" w794 {
                          tunnel: w793 -> [_ w800]
                          tunnel: w792 -> [_ w801]
                          frame #0 {
                          }
                          frame #1 {
                            n252 = Bundle(w801, w800) -> (w799:cluster{dbl, dbl})  [unwired: 1 in]
                            n253 = local write "Polar Display (T)"(w799) -> ()
                          }
                        }
                      }
                    }
                  }
                }
              }
            }
          }
          frame #1 {
            # "Zeile in Datei schreiben"
            # "Read and Save Devices"
            n254 = stacked-sequence {
              tunnel: [w829 _ _ _ _ _ _] -> w822
              tunnel: [w828 _ _ _ _ _ _] -> w821
              tunnel: [_ w842 _ _ _ _ _] -> w818
              tunnel: [_ w840 _ _ _ _ _] -> w817
              tunnel: [_ _ w852 _ _ _ _] -> w816
              tunnel: [_ _ w851 _ _ _ _] -> w815
              tunnel: [_ _ _ w863 _ _ _] -> w814
              tunnel: [_ _ _ 0.0 _ _ _] -> w813
              tunnel: [_ _ _ _ w869 _ _] -> w812
              tunnel: [_ _ _ _ _ _ w880] -> w804
              tunnel: [_ _ _ _ _ w875 _] -> w803
              tunnel: [_ _ _ _ _ w874 _] -> w802
              frame #0 {
                n255 = local read "LI 1"() -> (w827:bool)
                n256 = case shown="False" w827 {
                  tunnel: ["0" ("Antwort2") w836] -> w831
                  tunnel: ["0" ("Antwort1") w835] -> w830
                  frame #0 {
                  }
                  frame #1 {
                    n257 = local read "GPIB L 1"() -> (w834:string)
                    n258 = call "LI-Ansteuerung.vi"("Frage2"="OUTP? 4", "Frage1"="OUTP? 1", "address string"=w834) -> ("Antwort2"=w836:string, "Antwort1"=w835:string)
                  }
                }
                n259 = Fract/Exp String To Number(string=w831) -> (number=w828:dbl)  [unwired: 3 in, 1 out]
                n260 = Fract/Exp String To Number(string=w830) -> (number=w829:dbl)  [unwired: 3 in, 1 out]
              }
              frame #1 {
                n261 = local read "LI 2"() -> (w839:bool)
                n262 = case shown="False" w839 {
                  tunnel: [w844 w847] -> w841
                  tunnel: [w844 w846] -> w843
                  frame #0 {
                    w844 = "0" ("Antwort1")
                  }
                  frame #1 {
                    n263 = local read "GPIB L 2"() -> (w845:string)
                    n264 = call "LI-Ansteuerung.vi"("Frage2"="OUTP? 4", "Frage1"="OUTP? 1", "address string"=w845) -> ("Antwort2"=w847:string, "Antwort1"=w846:string)
                  }
                }
                n265 = Fract/Exp String To Number(string=w841) -> (number=w840:dbl)  [unwired: 3 in, 1 out]
                n266 = Fract/Exp String To Number(string=w843) -> (number=w842:dbl)  [unwired: 3 in, 1 out]
              }
              frame #2 {
                n267 = local read "LI 3"() -> (w850:bool)
                n268 = case shown="False" w850 {
                  tunnel: [w855 w858] -> w853
                  tunnel: [w855 w857] -> w854
                  frame #0 {
                    w855 = "0" ("Antwort1")
                  }
                  frame #1 {
                    n269 = local read "GPIB L 3"() -> (w856:string)
                    n270 = call "LI-Ansteuerung.vi"("Frage2"="OUTP? 4", "Frage1"="OUTP? 1", "address string"=w856) -> ("Antwort2"=w858:string, "Antwort1"=w857:string)
                  }
                }
                n271 = Fract/Exp String To Number(string=w854) -> (number=w852:dbl)  [unwired: 3 in, 1 out]
                n272 = Fract/Exp String To Number(string=w853) -> (number=w851:dbl)  [unwired: 3 in, 1 out]
              }
              frame #3 {
                n273 = local read "HP 1"() -> (w861:bool)
                n274 = case shown="True" w861 {
                  tunnel: [0.0 ("Voltage") w866] -> w863
                  frame #0 {
                  }
                  frame #1 {
                    n275 = local read "GPIB HP"() -> (w865:string)
                    n276 = call "HP-ReadVoltagev2.vi"("String"="meas:volt:dc? 250,0.001", "HP-Mulitmeter\nGPIB Address"=w865) -> ("Voltage"=w866:dbl)  [unwired: 9 in]
                  }
                }
              }
              frame #4 {
                n277 = local read "HP 2"() -> (w868:bool)
                n278 = case shown="True" w868 {
                  tunnel: [0.0 ("Voltage") w873] -> w869
                  frame #0 {
                  }
                  frame #1 {
                    n279 = local read "GPIB HP 2"() -> (w871:string)
                    n280 = call "HP-ReadVoltagev2.vi"("String"="meas:volt:dc? 200,0.001", "HP-Mulitmeter\nGPIB Address"=w871) -> ("Voltage"=w873:dbl)  [unwired: 9 in]
                  }
                }
              }
              frame #5 {
                n281 = local read "AH (2500)"() -> (w876:bool)
                n282 = case shown="False" w876 {
                  tunnel: [w877 w879] -> w875
                  tunnel: [w877 w878] -> w874
                  frame #0 {
                    w877 = 0.0 ("Voltage")
                  }
                  frame #1 {
                    n283 = call "AHRead2.vi"() -> ("loss"=w879:dbl, "capacitance"=w878:dbl)  [unwired: 8 in, 2 out]
                  }
                }
              }
              frame #6 {
                n284 = Get Date/Time In Seconds() -> (seconds since 1Jan1904=w881:timestamp)
                n285 = To Double Precision Float(number=w881) -> (double precision float=w880:dbl)
              }
            }
            n286 = Build Array(w824, w823, w822, w821, w818, w817, w815, w816, w814, w813, w812, w802, w803, w804) -> (w811:dbl[])
            n287 = Array To Spreadsheet String(array=w811, 3:"%f" ("format string")) -> (spreadsheet string=w820:string)  [unwired: 1 in]
            n288 = local read "Messfile Refnum"() -> (w805:refnum<file>)
            n289 = Set File Position(refnum=w805, from (0:start)=1, error in=w826) -> (refnum out=w807:refnum<file>, error out=w808:errorcluster)  [unwired: 1 in]
            n290 = Write to Text File(file (use dialog)=w807, text=w820, error in=w808) -> (refnum out=w810:refnum<file>, error out=w809:errorcluster)  [unwired: 1 in, 1 out]
            n291 = Flush File(refnum=w810, error in=w809) -> (error out=w825:errorcluster)  [unwired: 1 out]
          }
          frame #2 {
            n292 = local read "X Axis"() -> (w883:enum16{"B", "phi"})
            n293 = local read "Y Axis"() -> (w882:T1)
            n294 = local read "measured data"() -> (w887:dbl[][])
            n295 = Insert Into Array(array=w887, new element=w886) -> (w885:dbl[][])  [unwired: 2 in]
            n296 = case shown="0, Default" w884 {
              tunnel: w885 -> [w903 w917]
              tunnel: w882 -> [w905 w916]
              tunnel: w883 -> [w893 w915]
              frame #0 {
                n297 = Index Array(array=w903, index (col)=1 ("disabled index (col)")) -> (element=w898:dbl[])  [unwired: 1 in]
                n298 = Index Array(array=w903, index (col)=0 ("disabled index (col)")) -> (element=w897:dbl[])  [unwired: 1 in]
                n299 = Square(x=w898) -> (x^2=w900:dbl[])
                n300 = Square(x=w897) -> (x^2=w901:dbl[])
                n301 = Index Array(array=w903, index (col)=w905) -> (element=w892:dbl[])  [unwired: 1 in]
                n302 = Divide(x=w898, y=w897) -> (x/y=w889:dbl[])
                n303 = Add(x=w901, y=w900) -> (x+y=w899:dbl[])
                n304 = Inverse Tangent(1:w889) -> (0:w888:dbl[])
                n305 = Square Root(x=w899) -> (sqrt(x)=w890:dbl[])
                n306 = Divide(x=w888, y=3.141592653589793) -> (x/y=w895:dbl[])
                n307 = Multiply(x=w895, y=180) -> (x*y=w891:dbl[])
                n308 = case shown="\"phi\"" w893 {
                  tunnel: w892 -> [w908 w911]
                  tunnel: w891 -> [_ w910]
                  tunnel: w890 -> [w907 _]
                  frame #0 {
                    n309 = Bundle(w907, "measured data"=w908) -> (w906:cluster{dbl[], "measured data":dbl[]})  [unwired: 1 in]
                    n310 = local write "XY Graph"(w906) -> ()
                  }
                  frame #1 {
                    n311 = Bundle(w910, "measured data"=w911) -> (w909:cluster{dbl[], "measured data":dbl[]})  [unwired: 1 in]
                    n312 = local write "XY Graph"(w909) -> ()
                  }
                }
              }
              frame #1 {
                n313 = Index Array(array=w917, index (col)=w915) -> (element=w914:dbl[])  [unwired: 1 in]
                n314 = Index Array(array=w917, index (col)=w916) -> (element=w913:dbl[])  [unwired: 1 in]
                n315 = Bundle("measured data"=w914, "measured data"=w913) -> (w912:T2)  [unwired: 1 in]
                n316 = local write "XY Graph"(w912) -> ()
              }
            }
            n317 = local write "measured data"(w885) -> ()
          }
        }
        n318 = local read "Change\nPID\n(polar coordinates)"() -> (w685:bool)
        n319 = stacked-sequence {
          seq-local: [w696 _ _ _] -> [_ w707 w718 w728]
          seq-local: [w695 _ _ _] -> [_ _ w717 _]
          tunnel: w691 -> [w705 _ w720 _]
          tunnel: w690 -> [w704 _ w719 _]
          tunnel: w689 -> [w703 _ _ _]
          tunnel: [w696 _ _ _] -> w688
          tunnel: [_ _ w716 _] -> w687
          tunnel: w685 -> [_ w706 _ _]
          frame #0 {
            w699 = T9."HOLDING" ("y")
            n320 = call <userlib>:"Get Ramping Mode.vi"("Communications Config"=w705, "error in"=w703) -> ("Ramping Mode"=w701:T10, "error out"=w702:T5)  [unwired: 1 out]
            n321 = call <userlib>:"Get Ramping Mode.vi"("Communications Config"=w704, "error in"=w702) -> ("Ramping Mode"=w700:T10, "error out"=w695:T5)  [unwired: 1 out]
            n322 = Equal?(x=w700, y=w699) -> (x = y?=w698:bool)
            n323 = Equal?(x=w701, y=w699) -> (x = y?=w697:bool)
            n324 = And(x=w697, y=w698) -> (x .and. y?=w696:bool)
          }
          frame #1 {
            n325 = case shown="True" w707 {
              tunnel: w706 -> [_ w708]
              frame #0 {
              }
              frame #1 {
                n326 = case shown="True" w708 {
                  frame #0 {
                  }
                  frame #1 {
                    n327 = flat-sequence {
                      frame #0 {
                        n328 = call "SIM960Poff.vi"("off/on (0/1)"="0", "Port Num- PID"="1", "GPIB-Adress"="2") -> ()  [unwired: 9 in]
                      }
                      frame #1 {
                        n329 = call "SIM960Poff.vi"("off/on (0/1)"="0", "Port Num- PID"="3", "GPIB-Adress"="2") -> ()  [unwired: 9 in]
                      }
                    }
                  }
                }
                n330 = Wait (ms)(milliseconds to wait=u32 40000) -> ()  [unwired: 1 out]
              }
            }
          }
          frame #2 {
            n331 = case shown="True" w718 {
              tunnel: w720 -> [_ w727]
              tunnel: w719 -> [_ w726]
              tunnel: [w721 w723] -> w716
              tunnel: w717 -> [w721 w722]
              frame #0 {
              }
              frame #1 {
                w724 = u16 1 items=["RAMP", "PAUSE", "MANUAL UP", "MANUAL DOWN", "ZERO"] ("Ramping Mode")
                n332 = call <userlib>:"Set Ramping Mode.vi"("error in"=w722, "Ramping Mode"=w724, "Communications Config"=w727) -> ("error out"=w725:T5)
                n333 = call <userlib>:"Set Ramping Mode.vi"("error in"=w725, "Ramping Mode"=w724, "Communications Config"=w726) -> ("error out"=w723:T5)
              }
            }
          }
          frame #3 {
            n334 = case shown="True" w728 {
              frame #0 {
              }
              frame #1 {
                n335 = call <userlib>:"430_TCP_PSoff.vi"("IP Address"="111.111.111.2", "Switch Heater Control"=FALSE) -> ()  [unwired: 5 in, 2 out]
                n336 = call <userlib>:"430_TCP_PSoff.vi"("IP Address"="111.111.111.1", "Switch Heater Control"=FALSE) -> ()  [unwired: 5 in, 2 out]
              }
            }
          }
        }
      }
    }
  }
  n337 = Unbundle By Name(w8) -> ("Active Comm Interface"=w45:u16, "connection ID"=w44:refnum<k5>, "Serial Port"=w43:refnum<visa-resource-name>)
  n338 = Unbundle By Name(w7) -> ("Active Comm Interface"=w46:u16, "connection ID"=w42:refnum<k5>, "Serial Port"=w41:refnum<visa-resource-name>)
  n339 = case shown="0, Default" w46 {
    tunnel: w42 -> [w920 _ _]
    tunnel: [w919 w923 w924] -> w47
    tunnel: w41 -> [_ w922 _]
    tunnel: w6 -> [w918 w921 w924]
    frame #0 {
      n340 = call <userlib>:"430_TCP_Close.vi"("error in (no error)"=w918, "connection ID"=w920) -> ("error out"=w919:errorcluster)  [unwired: 1 out]
    }
    frame #1 {
      n341 = call <userlib>:"430_RS232_Close.vi"("error in (no error)"=w921, "VISA resource name"=w922) -> ("error out"=w923:errorcluster)  [unwired: 1 in]
    }
    frame #2 {
    }
  }
  n342 = case shown="0, Default" w45 {
    tunnel: w44 -> [w927 _ _]
    tunnel: w47 -> [w926 w930 w931]
    tunnel: [w925 w929 w931] -> w40
    tunnel: w43 -> [_ w928 _]
    frame #0 {
      n343 = call <userlib>:"430_TCP_Close.vi"("error in (no error)"=w926, "connection ID"=w927) -> ("error out"=w925:errorcluster)  [unwired: 1 out]
    }
    frame #1 {
      n344 = call <userlib>:"430_RS232_Close.vi"("error in (no error)"=w930, "VISA resource name"=w928) -> ("error out"=w929:errorcluster)  [unwired: 1 in]
    }
    frame #2 {
    }
  }
  "error out" <- w40
